vi "Main Responder.vi"(11 "CIFPluginManager in":refnum<class "CIFPluginManager.lvclass">) -> (0 "error out":errorcluster, 3 "Plugin Manager out":refnum<class "CIFPluginManager.lvclass">)   [LabVIEW 2021, in "CIFPluginManager.lvclass"]
uses:
  CIFPluginManager.lvclass
  gRPC/CIF_Manager_client/RPC Messages/cif_common_Empty.ctl
  CIFPluginManager.lvclass/CIFPluginManager.ctl
  <vilib>/Utility/miscctls.llb/LVMapReplaceAction.ctl
  gRPC/CIF_Manager_server/RPC Messages/cif_common_Empty.ctl
  CIFUtilities/CIFLogs/Typedef/Message Type.ctl
  gRPC/CIF_Manager_server/RPC Messages/cif_manager_UnregisterPluginLoaderResponse.ctl
  gRPC/CIF_Manager_server/RPC Messages/cif_manager_PluginTypeReply.ctl
  gRPC/CIF_Manager_server/RPC Messages/cif_manager_PluginType.ctl
  gRPC/CIF_Manager_server/RPC Messages/cif_common_ShortVersion.ctl
  gRPC/CIF_Manager_server/RPC Messages/cif_manager_PluginMetadata.ctl
  gRPC/CIF_Manager_server/RPC Messages/cif_channelcore_Channels.ctl
  gRPC/CIF_Manager_server/RPC Messages/cif_channelcore_Channel.ctl
  gRPC/CIF_Manager_server/RPC Messages/cif_channelcore_ChannelDirection.ctl
  gRPC/CIF_Manager_server/RPC Messages/cif_channelcore_ChannelPattern.ctl
  gRPC/CIF_Manager_server/RPC Messages/cif_manager_ErrorInfoList.ctl
  gRPC/CIF_Manager_server/RPC Messages/cif_manager_ErrorInfo.ctl
  gRPC/CIF_Manager_server/RPC Messages/cif_manager_FileData.ctl
  gRPC/CIF_Manager_server/RPC Messages/cif_manager_PluginInfoArray.ctl
  gRPC/CIF_Manager_server/RPC Messages/cif_manager_PluginInfo.ctl
  gRPC/CIF_Manager_server/RPC Messages/cif_plugincore_StatusData.ctl
  gRPC/CIF_Manager_server/RPC Messages/cif_plugincore_StatusData_PluginState.ctl
  gRPC/CIF_Manager_server/RPC Messages/cif_plugincore_TimingStatistics.ctl
  gRPC/CIF_Manager_server/RPC Messages/cif_common_TimingStats.ctl
  gRPC/CIF_Manager_server/RPC Messages/cif_plugincore_FifoStatistics.ctl
  gRPC/CIF_Manager_server/RPC Messages/cif_plugincore_Error.ctl
  gRPC/CIF_Manager_server/RPC Messages/cif_plugincore_MonitorDoubles.ctl
  gRPC/CIF_Manager_server/RPC Messages/cif_plugincore_MonitorU64.ctl
  gRPC/CIF_Manager_server/RPC Messages/cif_plugincore_MonitorI64.ctl
  gRPC/CIF_Manager_server/RPC Messages/cif_manager_LoaderInfo.ctl
  gRPC/CIF_Manager_server/RPC Messages/cif_manager_LoaderType.ctl
  CIFCore/Common/Typedef/Errors.ctl
  gRPC/CIF_Manager_server/RPC Messages/cif_manager_PluginInfoResponse.ctl
  gRPC/CIF_Manager_server/RPC Messages/cif_common_Status.ctl
  gRPC/CIF_Manager_server/RPC Messages/cif_manager_ClockStatusArray.ctl
  gRPC/CIF_Manager_server/RPC Messages/cif_manager_ClockStatus.ctl
  gRPC/CIF_Manager_server/RPC Messages/cif_manager_ClockConversion.ctl
  gRPC/CIF_Manager_server/RPC Messages/cif_manager_TimePair.ctl
  <vilib>/CIF Foundation/CIF Utilities/Time/Typedef/Timestamp Pair.ctl
  gRPC/CIF_Manager_server/RPC Messages/cif_manager_OrchReturn.ctl
  gRPC/CIF_Manager_server/RPC Messages/cif_manager_DestroyPluginLoaderResponse.ctl
  gRPC/CIF_Manager_server/RPC Messages/Get cif_manager_RegisterData.vi
  gRPC/CIF_Manager_server/RPC Messages/Set cif_common_Empty.vi
  gRPC/CIF_Manager_server/RPC Messages/Get cif_manager_RegisterPluginLoaderRequest.vi
  gRPC/CIF_Manager_server/RPC Messages/Set cif_manager_RegisterPluginLoaderResponse.vi
  gRPC/CIF_Manager_server/RPC Messages/Get cif_manager_UnregisterData.vi
  gRPC/CIF_Manager_server/RPC Messages/Get cif_manager_UnregisterPluginLoaderRequest.vi
  gRPC/CIF_Manager_server/RPC Messages/Set cif_manager_UnregisterPluginLoaderResponse.vi
  gRPC/CIF_Manager_server/RPC Messages/Get cif_manager_QueryTypeSettings.vi
  gRPC/CIF_Manager_server/RPC Messages/Set cif_manager_PluginTypeReply.vi
  gRPC/CIF_Manager_server/RPC Messages/Get cif_channelcore_ChannelFilter.vi
  gRPC/CIF_Manager_server/RPC Messages/Set cif_channelcore_Channels.vi
  gRPC/CIF_Manager_server/RPC Messages/Get cif_common_Empty.vi
  gRPC/CIF_Manager_server/RPC Messages/Set cif_common_Status.vi
  gRPC/CIF_Manager_server/RPC Messages/Get cif_manager_QuerySettings.vi
  gRPC/CIF_Manager_server/RPC Messages/Set cif_manager_ErrorInfoList.vi
  gRPC/CIF_Manager_server/RPC Messages/Set cif_manager_FileData.vi
  gRPC/CIF_Manager_server/RPC Messages/Set cif_manager_PluginInfoArray.vi
  gRPC/CIF_Manager_server/RPC Messages/Get cif_manager_PluginName.vi
  gRPC/CIF_Manager_server/RPC Messages/Set cif_manager_PluginInfoResponse.vi
  <vilib>/CIF Foundation/CIF Utilities/Errors/Append Error Location.vi
  gRPC/CIF_Manager_server/RPC Messages/Set cif_manager_ClockStatusArray.vi
  gRPC/CIF_Manager_server/RPC Messages/Get cif_manager_ClockUpdate.vi
  <vilib>/CIF Foundation/CIF Utilities/Time/SubVIs/Weighted Moving Average for Slope.vi
  <vilib>/CIF Foundation/CIF Utilities/DataTypes/Utilities/Valid Number.vi
  gRPC/CIF_Manager_server/RPC Messages/Get cif_manager_OrchConfig.vi
  gRPC/CIF_Manager_server/RPC Messages/Set cif_manager_OrchReturn.vi
  gRPC/CIF_Manager_server/RPC Messages/Get cif_manager_DestroyPluginLoaderRequest.vi
  gRPC/CIF_Manager_server/RPC Messages/Set cif_manager_DestroyPluginLoaderResponse.vi
  gRPC/CIF_Manager_server/RPC Messages/Get cif_manager_RegisterData.vi/2ed25e12-861d-4677-8ead-ace2906b2041.vi
  gRPC/CIF_Manager_server/RPC Messages/FlatToRichcif_manager_RegisterData.vi
  gRPC/CIF_Manager_server/RPC Messages/Set cif_common_Empty.vi/dcc74a39-081a-4bdd-860b-8ed792803c96.vi
  gRPC/CIF_Manager_server/RPC Messages/RichToFlatcif_common_Empty.vi
  gRPC/CIF_Manager_server/RPC Messages/Get cif_manager_RegisterPluginLoaderRequest.vi/2ed25e12-861d-4677-8ead-ace2906b2041.vi
  gRPC/CIF_Manager_server/RPC Messages/FlatToRichcif_manager_RegisterPluginLoaderRequest.vi
  gRPC/CIF_Manager_server/RPC Messages/Set cif_manager_RegisterPluginLoaderResponse.vi/dcc74a39-081a-4bdd-860b-8ed792803c96.vi
  gRPC/CIF_Manager_server/RPC Messages/RichToFlatcif_manager_RegisterPluginLoaderResponse.vi
  gRPC/CIF_Manager_server/RPC Messages/Get cif_manager_UnregisterData.vi/2ed25e12-861d-4677-8ead-ace2906b2041.vi
  gRPC/CIF_Manager_server/RPC Messages/FlatToRichcif_manager_UnregisterData.vi
  gRPC/CIF_Manager_server/RPC Messages/Get cif_manager_UnregisterPluginLoaderRequest.vi/2ed25e12-861d-4677-8ead-ace2906b2041.vi
  gRPC/CIF_Manager_server/RPC Messages/FlatToRichcif_manager_UnregisterPluginLoaderRequest.vi
  gRPC/CIF_Manager_server/RPC Messages/Set cif_manager_UnregisterPluginLoaderResponse.vi/dcc74a39-081a-4bdd-860b-8ed792803c96.vi
  gRPC/CIF_Manager_server/RPC Messages/RichToFlatcif_manager_UnregisterPluginLoaderResponse.vi
  gRPC/CIF_Manager_server/RPC Messages/Get cif_manager_QueryTypeSettings.vi/2ed25e12-861d-4677-8ead-ace2906b2041.vi
  gRPC/CIF_Manager_server/RPC Messages/FlatToRichcif_manager_QueryTypeSettings.vi
  gRPC/CIF_Manager_server/RPC Messages/Set cif_manager_PluginTypeReply.vi/dcc74a39-081a-4bdd-860b-8ed792803c96.vi
  gRPC/CIF_Manager_server/RPC Messages/RichToFlatcif_manager_PluginTypeReply.vi
  gRPC/CIF_Manager_server/RPC Messages/Get cif_channelcore_ChannelFilter.vi/2ed25e12-861d-4677-8ead-ace2906b2041.vi
  gRPC/CIF_Manager_server/RPC Messages/FlatToRichcif_channelcore_ChannelFilter.vi
  gRPC/CIF_Manager_server/RPC Messages/Set cif_channelcore_Channels.vi/dcc74a39-081a-4bdd-860b-8ed792803c96.vi
  gRPC/CIF_Manager_server/RPC Messages/RichToFlatcif_channelcore_Channels.vi
  gRPC/CIF_Manager_server/RPC Messages/Get cif_common_Empty.vi/2ed25e12-861d-4677-8ead-ace2906b2041.vi
  gRPC/CIF_Manager_server/RPC Messages/FlatToRichcif_common_Empty.vi
  gRPC/CIF_Manager_server/RPC Messages/Set cif_common_Status.vi/dcc74a39-081a-4bdd-860b-8ed792803c96.vi
  gRPC/CIF_Manager_server/RPC Messages/RichToFlatcif_common_Status.vi
  gRPC/CIF_Manager_server/RPC Messages/Get cif_manager_QuerySettings.vi/2ed25e12-861d-4677-8ead-ace2906b2041.vi
  gRPC/CIF_Manager_server/RPC Messages/FlatToRichcif_manager_QuerySettings.vi
  gRPC/CIF_Manager_server/RPC Messages/Set cif_manager_ErrorInfoList.vi/dcc74a39-081a-4bdd-860b-8ed792803c96.vi
  gRPC/CIF_Manager_server/RPC Messages/RichToFlatcif_manager_ErrorInfoList.vi
  gRPC/CIF_Manager_server/RPC Messages/Set cif_manager_FileData.vi/dcc74a39-081a-4bdd-860b-8ed792803c96.vi
  gRPC/CIF_Manager_server/RPC Messages/RichToFlatcif_manager_FileData.vi
  gRPC/CIF_Manager_server/RPC Messages/Set cif_manager_PluginInfoArray.vi/dcc74a39-081a-4bdd-860b-8ed792803c96.vi
  gRPC/CIF_Manager_server/RPC Messages/RichToFlatcif_manager_PluginInfoArray.vi
  gRPC/CIF_Manager_server/RPC Messages/Get cif_manager_PluginName.vi/2ed25e12-861d-4677-8ead-ace2906b2041.vi
  gRPC/CIF_Manager_server/RPC Messages/FlatToRichcif_manager_PluginName.vi
  gRPC/CIF_Manager_server/RPC Messages/Set cif_manager_PluginInfoResponse.vi/dcc74a39-081a-4bdd-860b-8ed792803c96.vi
  gRPC/CIF_Manager_server/RPC Messages/RichToFlatcif_manager_PluginInfoResponse.vi
  gRPC/CIF_Manager_server/RPC Messages/Set cif_manager_ClockStatusArray.vi/dcc74a39-081a-4bdd-860b-8ed792803c96.vi
  gRPC/CIF_Manager_server/RPC Messages/RichToFlatcif_manager_ClockStatusArray.vi
  gRPC/CIF_Manager_server/RPC Messages/Get cif_manager_ClockUpdate.vi/2ed25e12-861d-4677-8ead-ace2906b2041.vi
  gRPC/CIF_Manager_server/RPC Messages/FlatToRichcif_manager_ClockUpdate.vi
  <vilib>/Analysis/3filter.llb/Savitzky-Golay Filter.vi
  <vilib>/Analysis/3filter.llb/Savitzky-Golay Filter (DBL).vi
  gRPC/CIF_Manager_server/RPC Messages/Get cif_manager_OrchConfig.vi/2ed25e12-861d-4677-8ead-ace2906b2041.vi
  gRPC/CIF_Manager_server/RPC Messages/FlatToRichcif_manager_OrchConfig.vi
  gRPC/CIF_Manager_server/RPC Messages/Set cif_manager_OrchReturn.vi/dcc74a39-081a-4bdd-860b-8ed792803c96.vi
  gRPC/CIF_Manager_server/RPC Messages/RichToFlatcif_manager_OrchReturn.vi
  gRPC/CIF_Manager_server/RPC Messages/Get cif_manager_DestroyPluginLoaderRequest.vi/2ed25e12-861d-4677-8ead-ace2906b2041.vi
  gRPC/CIF_Manager_server/RPC Messages/FlatToRichcif_manager_DestroyPluginLoaderRequest.vi
  gRPC/CIF_Manager_server/RPC Messages/Set cif_manager_DestroyPluginLoaderResponse.vi/dcc74a39-081a-4bdd-860b-8ed792803c96.vi
  gRPC/CIF_Manager_server/RPC Messages/RichToFlatcif_manager_DestroyPluginLoaderResponse.vi
  <vilib>/gRPC/LabVIEW gRPC Library/Shared/TranslateGrpcError.vi
  gRPC/CIF_Manager_server/RPC Messages/FlatToRichcif_common_ShortVersion.vi
  gRPC/CIF_Manager_server/RPC Messages/FlatToRichcif_manager_LoaderInfoFull.vi
  gRPC/CIF_Manager_server/RPC Messages/RichToFlatcif_manager_PluginType.vi
  gRPC/CIF_Manager_server/RPC Messages/RichToFlatcif_channelcore_Channel.vi
  gRPC/CIF_Manager_server/RPC Messages/RichToFlatcif_manager_ErrorInfo.vi
  gRPC/CIF_Manager_server/RPC Messages/RichToFlatcif_manager_PluginInfo.vi
  gRPC/CIF_Manager_server/RPC Messages/RichToFlatcif_manager_ClockStatus.vi
  gRPC/CIF_Manager_server/RPC Messages/FlatToRichcif_manager_TimePair.vi
  gRPC/CIF_Manager_server/RPC Messages/RichToFlatcif_common_ShortVersion.vi
  gRPC/CIF_Manager_server/RPC Messages/RichToFlatcif_manager_PluginMetadata.vi
  gRPC/CIF_Manager_server/RPC Messages/RichToFlatcif_plugincore_StatusData.vi
  gRPC/CIF_Manager_server/RPC Messages/RichToFlatcif_manager_LoaderInfo.vi
  gRPC/CIF_Manager_server/RPC Messages/RichToFlatcif_manager_ClockConversion.vi
  gRPC/CIF_Manager_server/RPC Messages/RichToFlatcif_plugincore_TimingStatistics.vi
  gRPC/CIF_Manager_server/RPC Messages/RichToFlatcif_plugincore_FifoStatistics.vi
  gRPC/CIF_Manager_server/RPC Messages/RichToFlatcif_plugincore_Error.vi
  gRPC/CIF_Manager_server/RPC Messages/RichToFlatcif_plugincore_MonitorDoubles.vi
  gRPC/CIF_Manager_server/RPC Messages/RichToFlatcif_plugincore_MonitorU64.vi
  gRPC/CIF_Manager_server/RPC Messages/RichToFlatcif_plugincore_MonitorI64.vi
  gRPC/CIF_Manager_server/RPC Messages/RichToFlatcif_manager_TimePair.vi
  gRPC/CIF_Manager_server/RPC Messages/RichToFlatcif_common_TimingStats.vi
  <vilib>/gRPC/LabVIEW gRPC Library/Server API/Server/Get Server DLL Path.vi
  <vilib>/Utility/error.llb/Error Cluster From Error Code.vi
  <vilib>/gRPC/LabVIEW gRPC Library/Server API/Message Requests/Complete Call.vi
  <vilib>/Analysis/baseanly.llb/Std Deviation and Variance.vi
  <vilib>/Analysis/6fits.llb/Linear Fit.vi
  <vilib>/regexp/Match Regular Expression.xnode
  CIFUtilities/CIFLogs/CIFLogs.lvlib
  gRPC/CIF_Manager_Client_Wrapper/CIFManagerClientWrapper.lvlib
  gRPC/CIF_Manager_client/CIF_Manager_client.lvlib
  gRPC/CIF_Manager_server/RPC Service/Manager/Manager.lvclass
  <vilib>/CIF Foundation/CIF Utilities/Time/Time_CIF_U.lvlib
  CIFCore/Grpc/CIFCoreWrapper/CIFCoreWrapper.lvlib
  CIFUtilities/CIFConfigurationFile/CIF Configuration File.lvlib
  gRPC/CIF_Manager_server/CIF_Manager_server.lvlib
  CIFPluginLoader/gRPC/CIF_Plugin_Loader_Client_Wrapper/CIFPluginLoaderClientWrapper.lvlib
  CIFCore/Common/CIFCoreCommon.lvlib
  CIFUtilities/Scripting/Orchestration/Python/Python Orchestration.lvlib
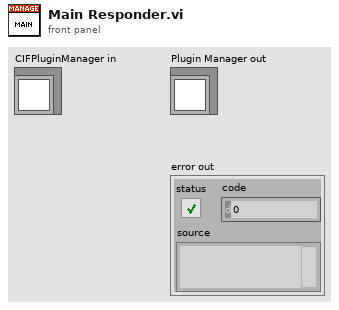
[diagram p1: front panel]
types:
  T1 = typedef "CIF_Manager_client.lvlib/cif_common_Empty.ctl" = cluster{"void":string}
  T2 = typedef "LVMapReplaceAction.ctl" = enum32{"Modify Entry only if found", "Add or Modify Entry", "Delete Entry"}
  T3 = typedef "CIF_Manager_server.lvlib/cif_common_Empty.ctl" = cluster{"void":string}
  T4 = typedef "CIFLogs.lvlib/Message Type.ctl" = enum16{"Error", "Information", "Print Terminal", "Configuration"}
  T5 = typedef "CIF_Manager_server.lvlib/cif_manager_UnregisterPluginLoaderResponse.ctl" = cluster{"void":string}
  T6 = typedef "CIF_Manager_server.lvlib/cif_manager_PluginTypeReply.ctl" = cluster{"plugin_types":T7[]}
  T7 = typedef "CIF_Manager_server.lvlib/cif_manager_PluginType.ctl" = cluster{"plugin_type":string, "plugin_version":T8, "plugin_metadata":T9, "relative_path":string[]}
  T8 = typedef "CIF_Manager_server.lvlib/cif_common_ShortVersion.ctl" = cluster{"major":u32, "minor":u32, "fix":u32}
  T9 = typedef "CIF_Manager_server.lvlib/cif_manager_PluginMetadata.ctl" = cluster{"description":string, "history":string, "author":string}
  T10 = typedef "CIF_Manager_server.lvlib/cif_channelcore_Channels.ctl" = cluster{"channels":T11[]}
  T11 = typedef "CIF_Manager_server.lvlib/cif_channelcore_Channel.ctl" = cluster{"name":string, "direction":T12, "type":string, "custom_config":u8[], "connected":bool, "connected_name":string, "forced":bool, "channel_pattern":T13}
  T12 = typedef "CIF_Manager_server.lvlib/cif_channelcore_ChannelDirection.ctl" = enum32{"CHANNELDIRECTION_UNKNOWN", "CHANNELDIRECTION_PUBLISHER", "CHANNELDIRECTION_SUBSCRIBER"}
  T13 = typedef "CIF_Manager_server.lvlib/cif_channelcore_ChannelPattern.ctl" = enum32{"CHANNELPATTERN_UNKNOWN", "CHANNELPATTERN_TAG", "CHANNELPATTERN_FIFO", "CHANNELPATTERN_MULTIFIFO", "CHANNELPATTERN_BACKPRESSUREFIFO"}
  T14 = typedef "CIF_Manager_server.lvlib/cif_manager_ErrorInfoList.ctl" = cluster{"error_info":T15[]}
  T15 = typedef "CIF_Manager_server.lvlib/cif_manager_ErrorInfo.ctl" = cluster{"error_status":bool, "error_code":i32, "plugin":string, "time":string, "message":string, "location":string}
  T16 = typedef "CIF_Manager_server.lvlib/cif_manager_FileData.ctl" = cluster{"data":string}
  T17 = typedef "CIF_Manager_server.lvlib/cif_manager_PluginInfoArray.ctl" = cluster{"plugin_info":T18[]}
  T18 = typedef "CIF_Manager_server.lvlib/cif_manager_PluginInfo.ctl" = cluster{"plugin_name":string, "plugin_type":string, "grpc_port":i32, "plugin_version":T8, "status":T19, "loader_info":T28}
  T19 = typedef "CIF_Manager_server.lvlib/cif_plugincore_StatusData.ctl" = cluster{"state":T20, "timing_statistics":T21, "fifo_statistics":T23, "error":T24, "monitor_doubles":T25, "monitor_u64s":T26, "monitor_i64s":T27}
  T20 = typedef "CIF_Manager_server.lvlib/cif_plugincore_StatusData_PluginState.ctl" = enum32{"PLUGINSTATE_UNKNOWN", "PLUGINSTATE_CREATING", "PLUGINSTATE_LISTENING", "PLUGINSTATE_RUNNING", "PLUGINSTATE_CLEANINGUP", "PLUGINSTATE_DESTROYING"}
  T21 = typedef "CIF_Manager_server.lvlib/cif_plugincore_TimingStatistics.ctl" = cluster{"period":T22, "wake_error":T22, "execute":T22, "housekeep":T22, "idle":T22, "cleanup":T22, "custom_1":T22, "custom_2":T22}
  T22 = typedef "CIF_Manager_server.lvlib/cif_common_TimingStats.ctl" = cluster{"max":i64, "min":i64, "avg":dbl}
  T23 = typedef "CIF_Manager_server.lvlib/cif_plugincore_FifoStatistics.ctl" = cluster{"from_t0":T22, "from_previous_plugin":T22, "output_error":T22}
  T24 = typedef "CIF_Manager_server.lvlib/cif_plugincore_Error.ctl" = cluster{"status":bool, "code":i32}
  T25 = typedef "CIF_Manager_server.lvlib/cif_plugincore_MonitorDoubles.ctl" = cluster{"double_1":dbl, "double_2":dbl, "double_3":dbl, "double_4":dbl}
  T26 = typedef "CIF_Manager_server.lvlib/cif_plugincore_MonitorU64.ctl" = cluster{"u64_1":u64, "u64_2":u64, "u64_3":u64, "u64_4":u64}
  T27 = typedef "CIF_Manager_server.lvlib/cif_plugincore_MonitorI64.ctl" = cluster{"i64_1":i64, "i64_2":i64, "i64_3":i64, "i64_4":i64}
  T28 = typedef "CIF_Manager_server.lvlib/cif_manager_LoaderInfo.ctl" = cluster{"loader_type":T29, "loader_name":string}
  T29 = typedef "CIF_Manager_server.lvlib/cif_manager_LoaderType.ctl" = enum32{"LOADERTYPE_UNKNOWN", "LOADERTYPE_LABVIEW"}
  T30 = typedef "CIFCoreCommon.lvlib/Errors.ctl" = enum16{"Invalid Clock ID", "Long Sleep", "gRPC Server Not Found", "Config Parse", "Timestamp Wrap", "Delayed Execution", "Duplicate Channel", "Missing Channel", "Incorrect Type", "Flatten Error", "Unflatten Data", "Unique Name", "Plugin Not Found", "Plugin Type Not Found", "Plugin Version Not Found", "Manager Not Found", "Numerical Issue", "Time Jump", "Clock ID Match", "Channel Length", "Plugin Connection", "gRPC Server Connection", "PPL Name Match", "Build", "Config Log Parse", "Plugin Load", "UI Subpanel Load", "Python Name", "Invalid Name", "Unable to Change Ch Buffer", "Failed Kill", "Failed SysExec", "Function Not Implemented", "Load Timeout"}
  T31 = typedef "CIF_Manager_server.lvlib/cif_manager_PluginInfoResponse.ctl" = cluster{"plugin_info":T18, "status":T32}
  T32 = typedef "CIF_Manager_server.lvlib/cif_common_Status.ctl" = cluster{"code":i32, "message":string}
  T33 = typedef "CIF_Manager_server.lvlib/cif_manager_ClockStatusArray.ctl" = cluster{"clocks_status":T34[]}
  T34 = typedef "CIF_Manager_server.lvlib/cif_manager_ClockStatus.ctl" = cluster{"clock_conversion":T35, "error_mean":i64, "error_std_dev":i64}
  T35 = typedef "CIF_Manager_server.lvlib/cif_manager_ClockConversion.ctl" = cluster{"clock_id":u32, "last_reset":i64, "slope":dbl, "offset_pair":T36, "clock_name":string}
  T36 = typedef "CIF_Manager_server.lvlib/cif_manager_TimePair.ctl" = cluster{"system_time":i64, "external_time":i64}
  T37 = typedef "Time_CIF_U.lvlib/Timestamp Pair.ctl" = cluster{"System Time":i64, "External Time":i64}
  T38 = typedef "CIF_Manager_server.lvlib/cif_manager_OrchReturn.ctl" = cluster{"orchestration_script":string, "status":T32}
  T39 = typedef "CIF_Manager_server.lvlib/cif_manager_DestroyPluginLoaderResponse.ctl" = cluster{"status":T32}
  T40 = typedef "grpc-lvsupport-release.lvlib/grpcId.ctl" = u64
  T41 = typedef "CIF_Manager_server.lvlib/cif_manager_RegisterData.ctl" = cluster{"plugin_name":string, "grpc_port":i32, "plugin_version":T8}
  T42 = typedef "CIFPluginManager.lvclass/Plugin Management Data Map.ctl" = map{string, T43}
  T43 = typedef "CIFPluginManager.lvclass/Plugin Management Data.ctl" = cluster{"Unique Name":string, "Plugin Type":string, "gRPC Port":i32, "gRPC ID":T40, "Loader Type":T44, "Loader":string, "Version":T45, "Load Timestamp":i64, "Unload Timestamp":i64, "Unloading":bool, "Ready for removal":bool, "status":T19, "channels":T10}
  T44 = typedef "CIFPluginManager.lvclass/Loader Type.ctl" = enum16{"LabVIEW"}
  T45 = typedef "CIFCoreCommon.lvlib/Version.ctl" = cluster{"Major":i32, "Minor":i32, "Fix":i32, "Build":i32}
  T46 = typedef "CIF_Manager_server.lvlib/cif_manager_RegisterPluginLoaderRequest.ctl" = cluster{"loader_info":T47}
  T47 = typedef "CIF_Manager_server.lvlib/cif_manager_LoaderInfoFull.ctl" = cluster{"loader_type":T29, "loader_name":string, "grpc_port":i32, "pid":u32}
  T48 = typedef "CIFPluginManager.lvclass/Loader Map.ctl" = map{string, T49}
  T49 = typedef "CIFPluginManager.lvclass/Loaders.ctl" = cluster{"Loader Type":T44, "grpc_port":i32, "pid":u32, "gRPC ID":T40, "Load Timestamp":i64, "Unloading":bool, "Ready for removal":bool, "Unload Timestamp":i64}
  T50 = typedef "CIF_Manager_server.lvlib/cif_manager_UnregisterData.ctl" = cluster{"plugin_name":string, "unregister_channels":string[]}
  T51 = typedef "CIF_Manager_server.lvlib/cif_manager_UnregisterPluginLoaderRequest.ctl" = cluster{"loader_name":string}
  T52 = typedef "CIF_Manager_server.lvlib/cif_manager_QueryTypeSettings.ctl" = cluster{"reload":bool}
  T53 = typedef "CIFPluginManager.lvclass/Discovered Plugin Map.ctl" = map{string, T54[]}
  T54 = typedef "CIFPluginManager.lvclass/Discovered Plugin.ctl" = cluster{"Filename":string, "Plugin Type":string, "Qualified name":string, "Version":T45, "Plugin Metadata":T55, "Loader Type":T44, "File Path":string, "Relative Path":string[]}
  T55 = typedef "CIFPluginManager.lvclass/Plugin Metadata.ctl" = cluster{"Description":string, "History":string, "Author":string}
  T56 = typedef "CIF_Manager_server.lvlib/cif_channelcore_ChannelFilter.ctl" = cluster{"name_regex":string, "direction":T12, "direction_filter":bool, "type_regex":string, "forced":bool, "forced_filter":bool}
  T57 = typedef "CIF_Manager_client.lvlib/cif_common_Status.ctl" = cluster{"code":i32, "message":string}
  T58 = typedef "CIF_Manager_server.lvlib/cif_manager_QuerySettings.ctl" = cluster{"query_all":bool}
  T59 = typedef "CIFLogs.lvlib/Error Message.ctl" = cluster{"error":bool, "code":i32, "Message":string, "Location":string, "Plugin":string, "Time":string}
  T60 = typedef "CIFLogs.lvlib/Log Info.ctl" = cluster{"size (bytes)":i64, "Last Timestamp":string}
  T61 = typedef "CIF_Manager_server.lvlib/cif_manager_PluginName.ctl" = cluster{"plugin_name":string}
  T62 = typedef "Time_CIF_U.lvlib/Clock History Map.ctl" = map{u8, T63}
  T63 = typedef "Time_CIF_U.lvlib/Clock History.ctl" = cluster{"System Clock":i64[], "External Clock":i64[], "Last Reset Time":i64, "slope":dbl, "1/slope":dbl, "Offset Pair":T37, "Name":string}
  T64 = typedef "Time_CIF_U.lvlib/Clock Conversion.ctl" = cluster{"ClockID":u8, "Last Reset":i64, "Offset Pair":T37, "Slope":dbl, "1/Slope":dbl, "Name":string}
  T65 = typedef "Time_CIF_U.lvlib/Clock Error Statistics.ctl" = cluster{"mean":i64, "standard deviation":i64}
  T66 = typedef "CIF_Manager_server.lvlib/cif_manager_ClockUpdate.ctl" = cluster{"clock_id":u32, "timestamp_pair":T36, "reinit":bool, "clock_name":string}
  T67 = typedef "CIF_Manager_server.lvlib/cif_manager_OrchConfig.ctl" = cluster{"start_timestamp":u64, "create_file":bool, "orchestration_language":T68, "filename":string, "default_ip":string}
  T68 = typedef "CIF_Manager_server.lvlib/cif_manager_OrchestrationLanguage.ctl" = enum32{"ORCHESTRATIONLANGUAGE_UNKNOWN", "ORCHESTRATIONLANGUAGE_PYTHON"}
  T69 = typedef "CIF_Manager_server.lvlib/cif_manager_DestroyPluginLoaderRequest.ctl" = cluster{"loader_name":string}
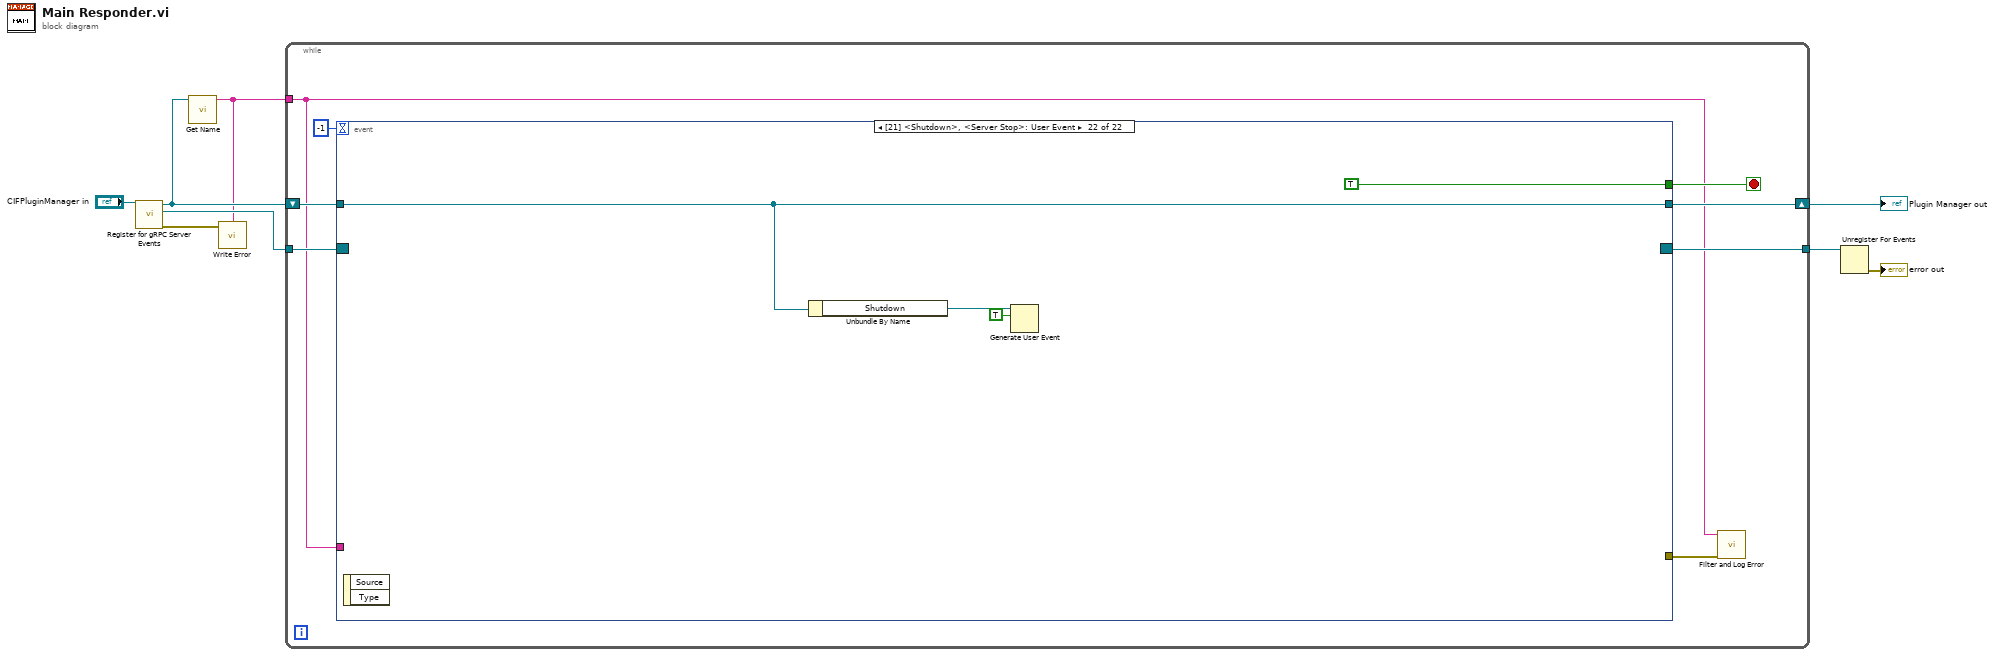
[diagram p0: block diagram]
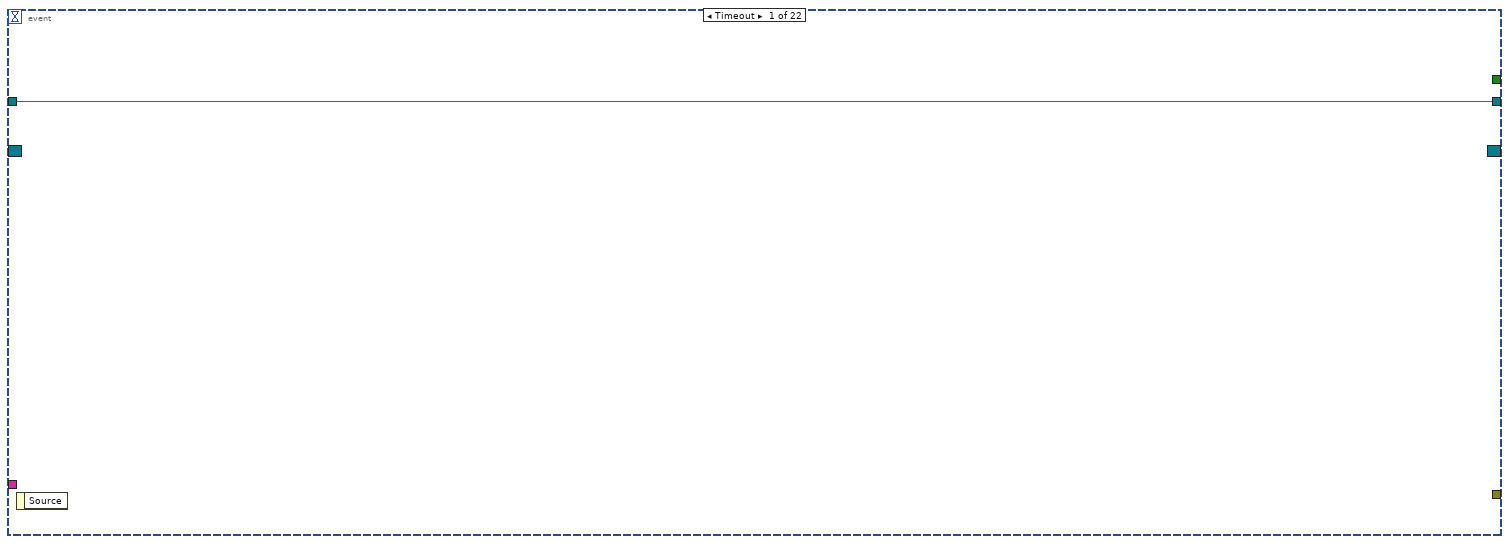
[diagram p2: hidden frame]
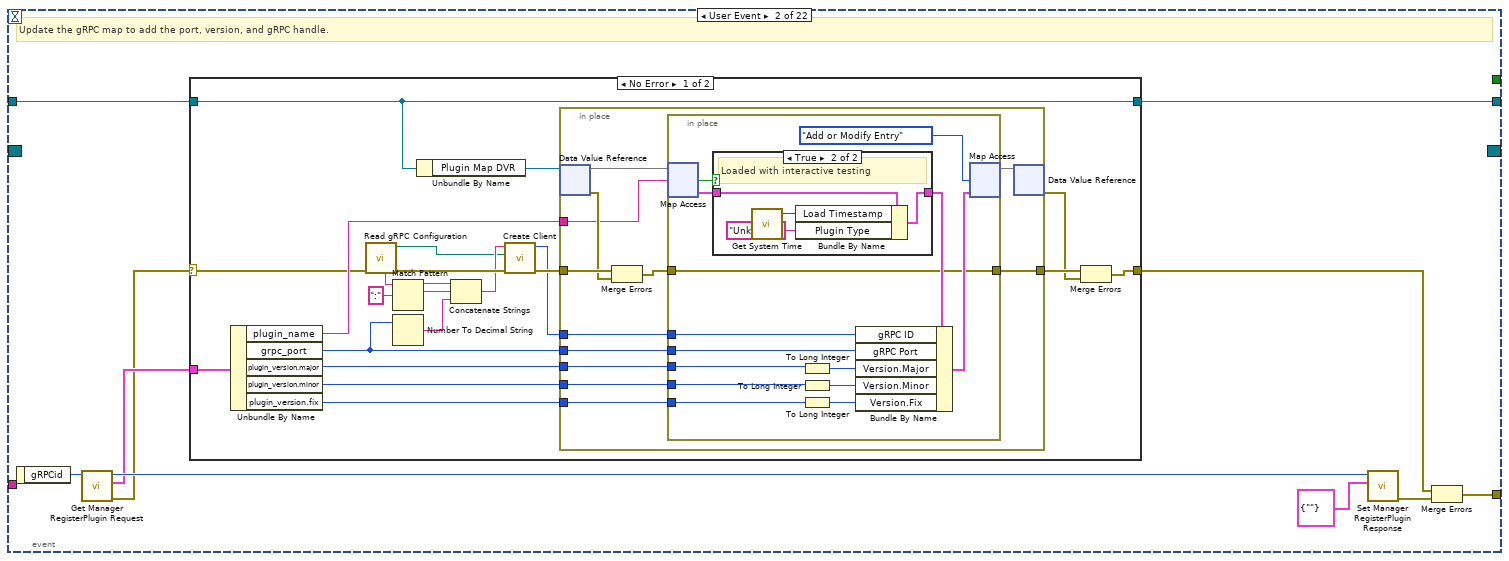
[diagram p3: hidden frame]
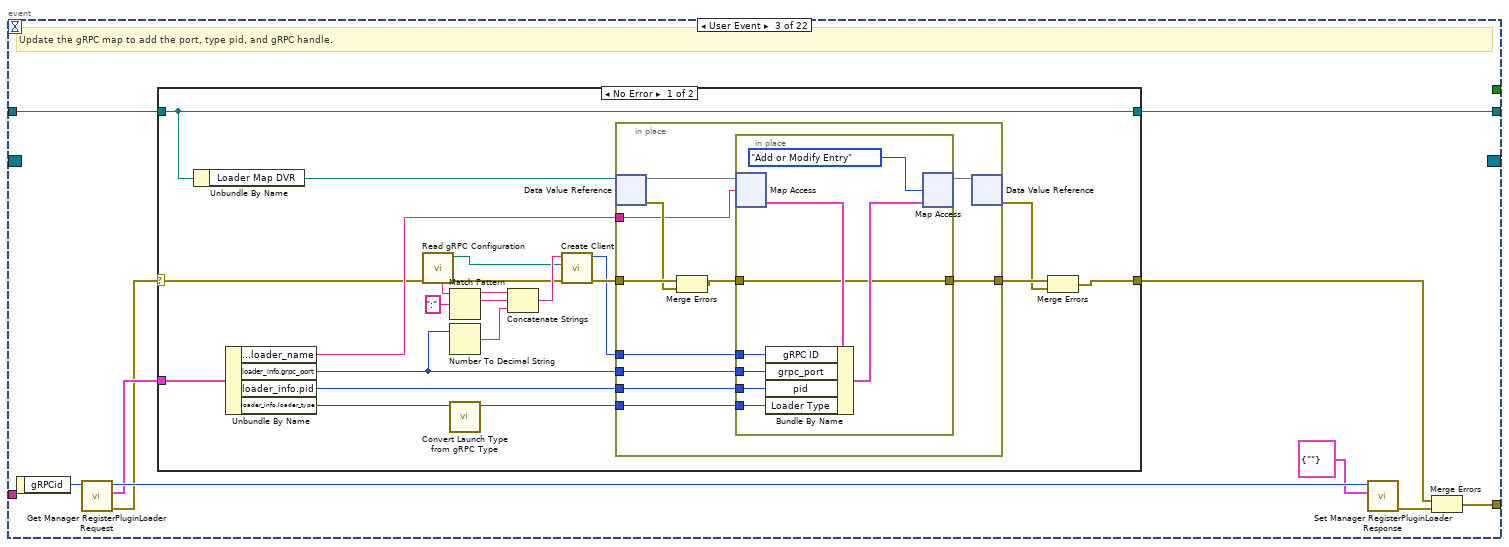
[diagram p6: hidden frame]
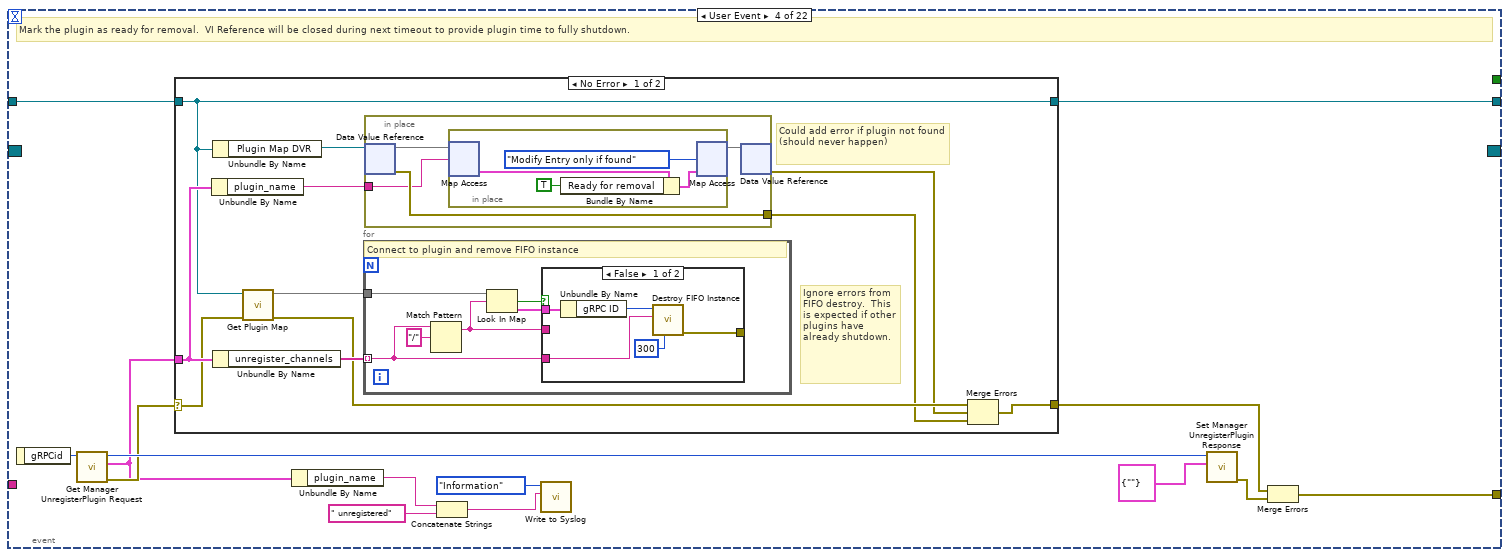
[diagram p8: hidden frame]
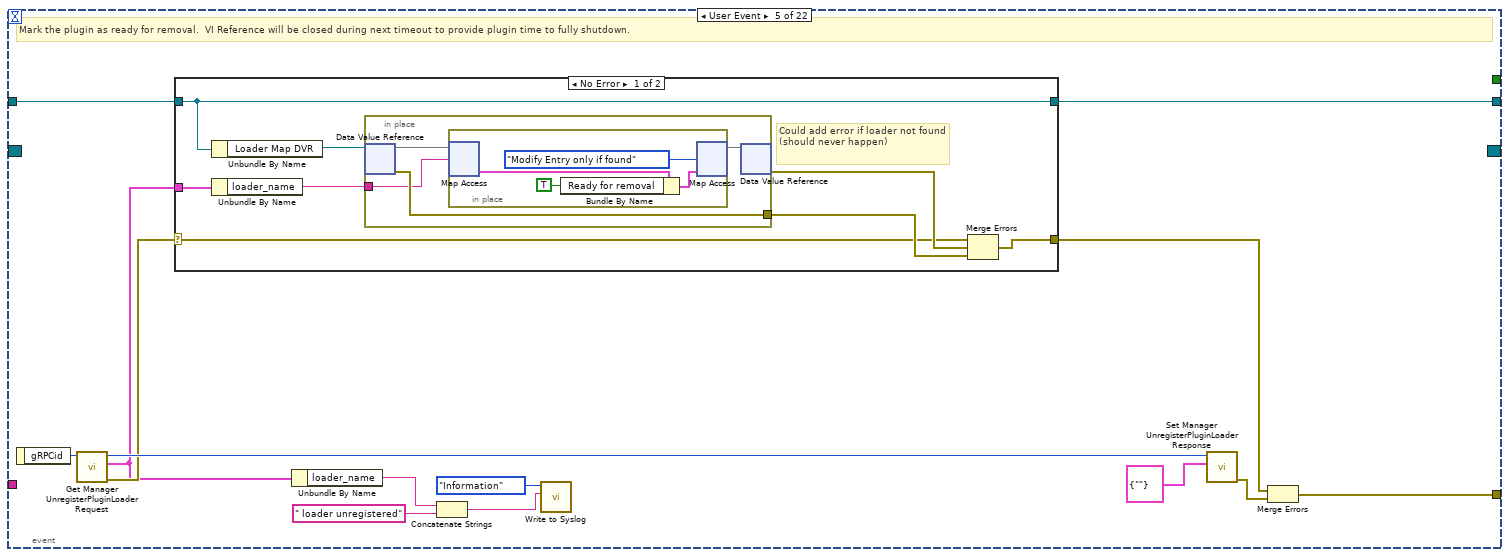
[diagram p11: hidden frame]
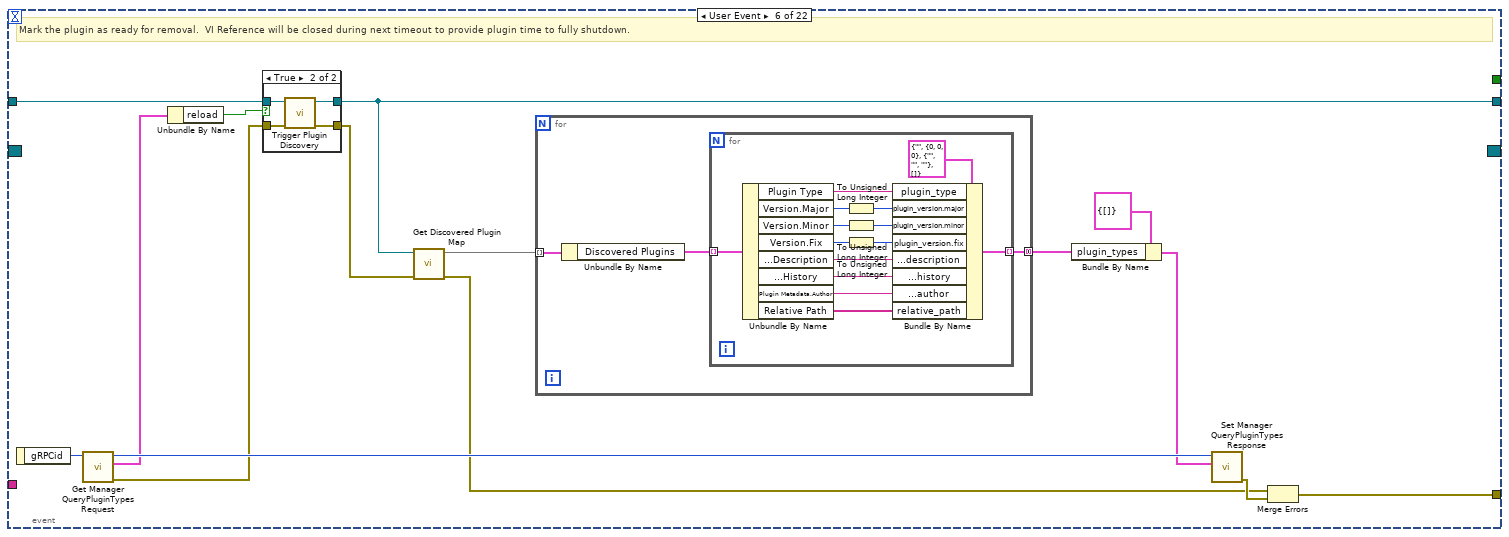
[diagram p13: hidden frame]
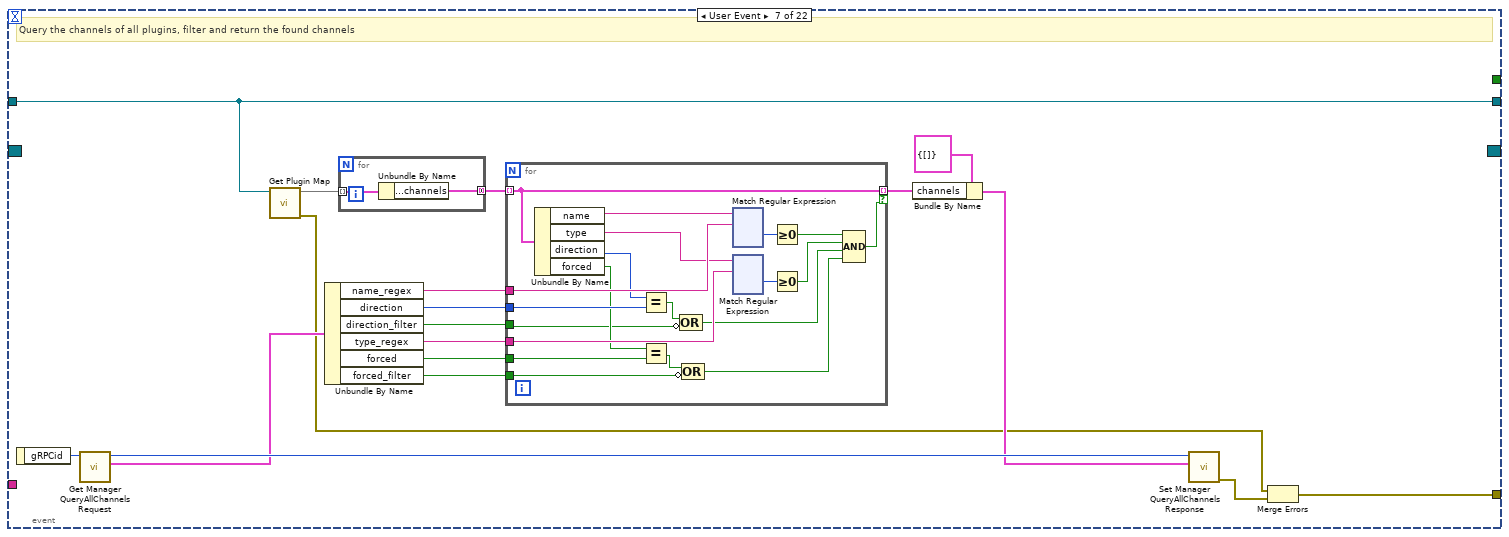
[diagram p15: hidden frame]
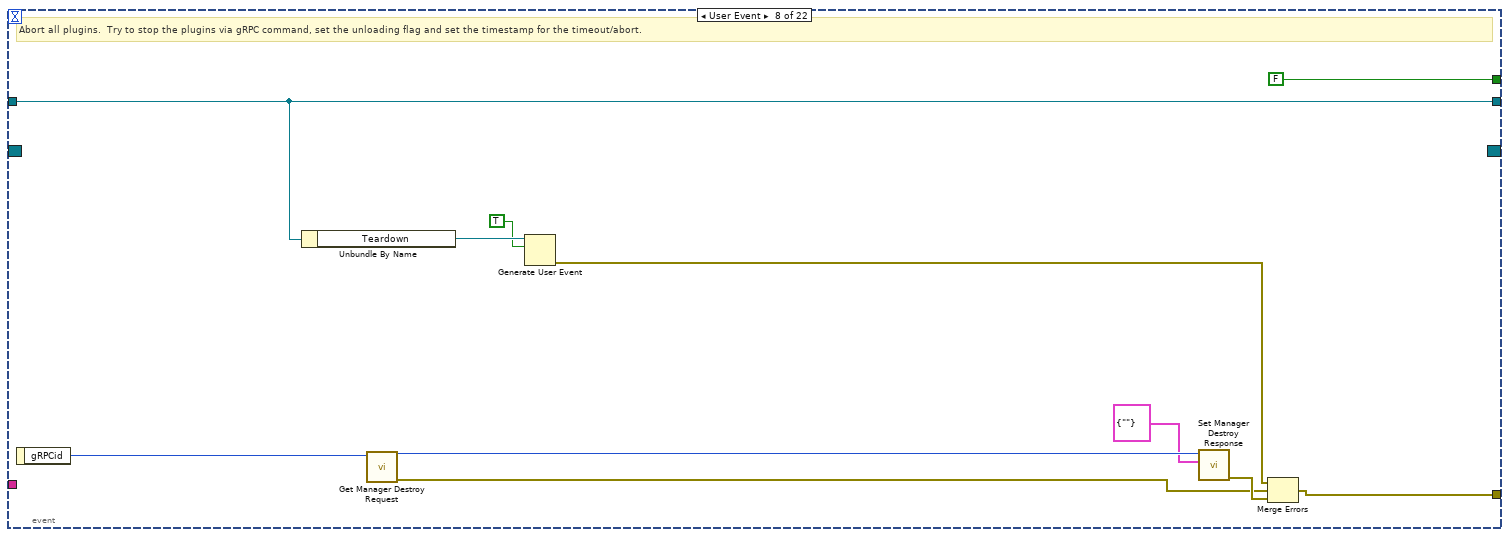
[diagram p16: hidden frame]
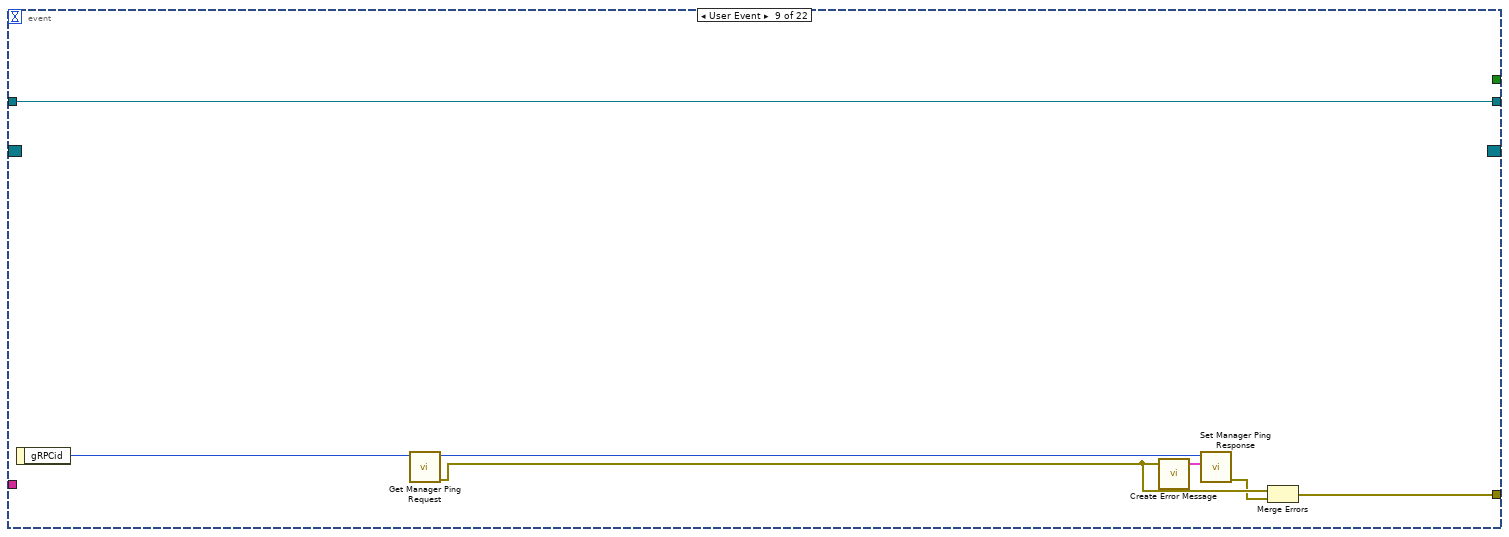
[diagram p17: hidden frame]
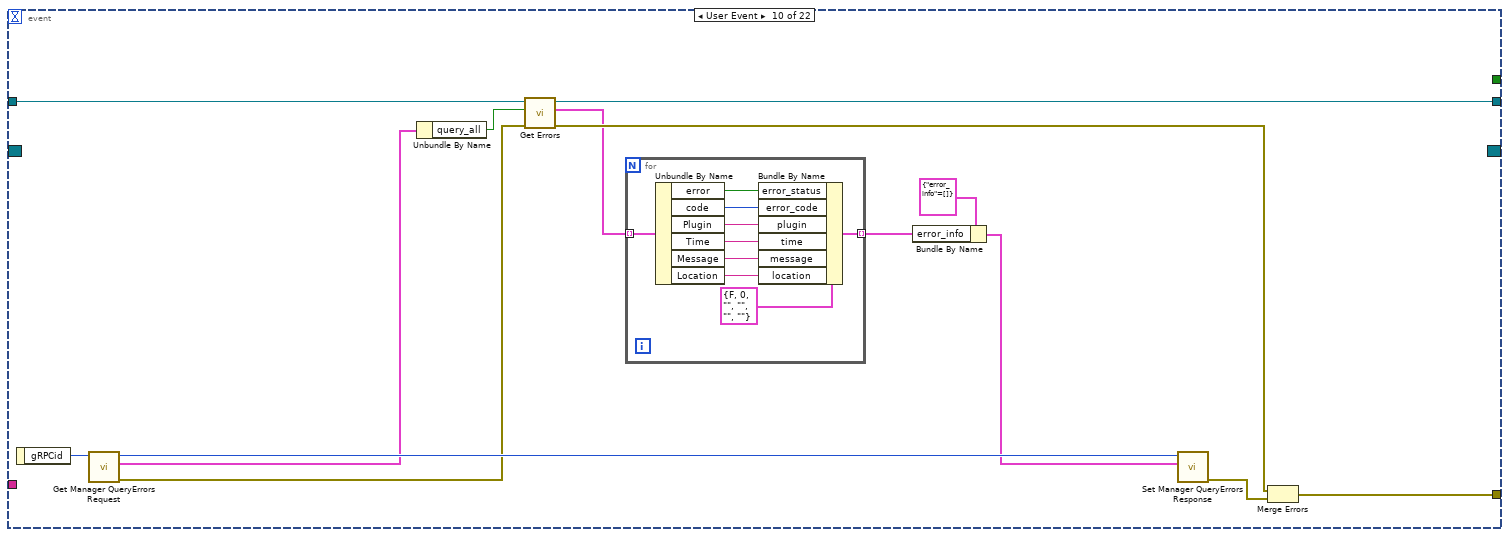
[diagram p18: hidden frame]
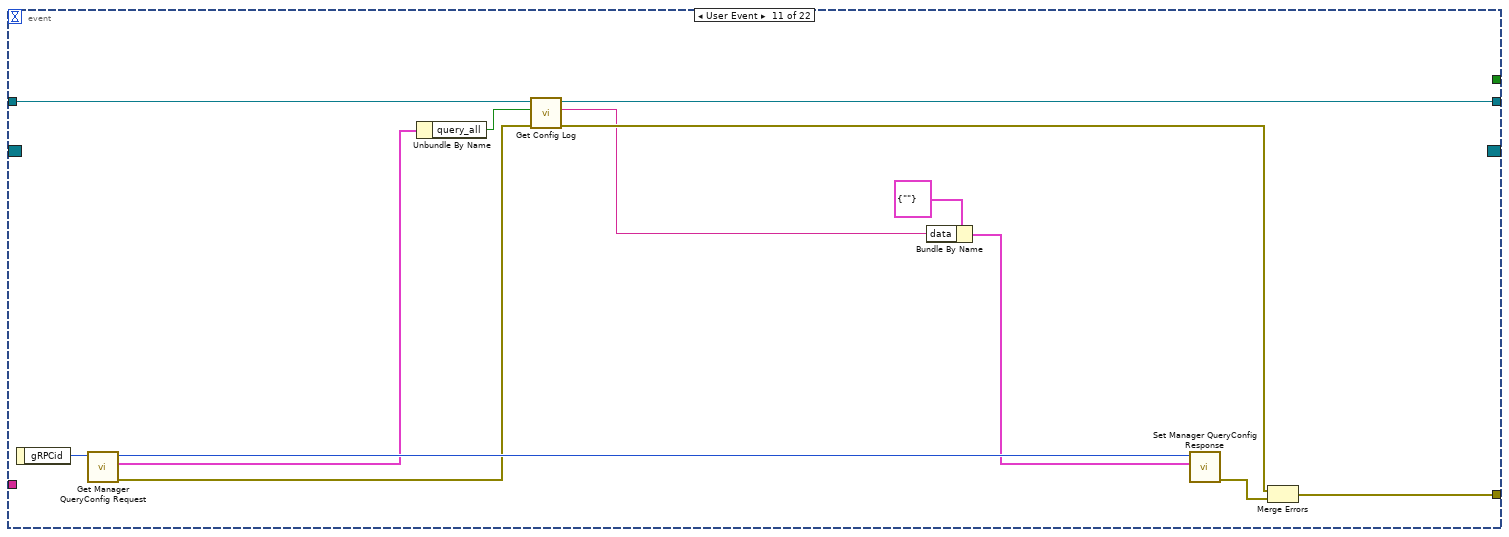
[diagram p19: hidden frame]
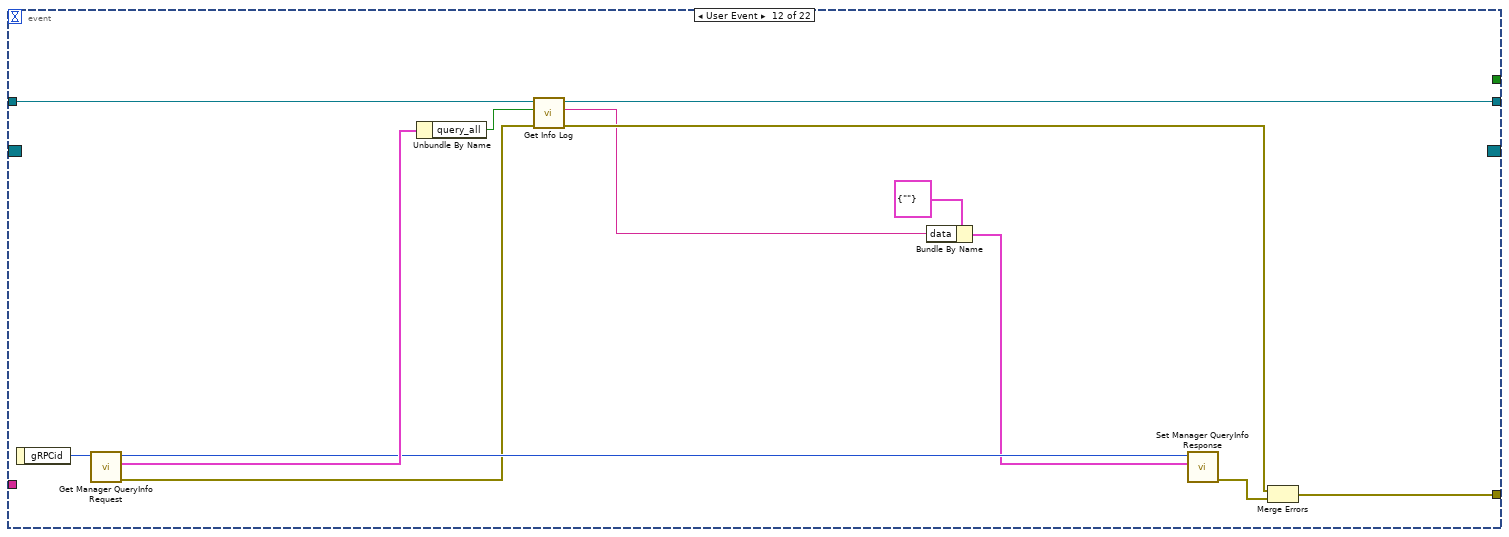
[diagram p20: hidden frame]
diagram:
  n1 = call "Register for gRPC Server Events.vi"("Plugin Manager in"="CIFPluginManager in") -> ("error out"=w8:errorcluster, "Event Registration Refnum"=w3:refnum<event-registration>, "Plugin Manager out"=w2:refnum<class "CIFPluginManager.lvclass">)  [unwired: 8 in]
  n2 = call "Get Name.vi"("CIFPluginManager in"=w2) -> ("Name"=w1:string)  [unwired: 10 in]
  n3 = call "Write Error.vi"("error in (no error)"=w8, "Plugin Name"=w1) -> ()  [unwired: 2 in, 1 out]
  n4 = while {
    tunnel: [w15] -> w6
    shift-right: [w14] -> w5
    shift-left: w2 -> [w16]
    tunnel: w3 -> [w11]
    tunnel: w1 -> [w9]
    stop <- w10 stop-if-true
    n5 = event shown="[21] <Shutdown>, <Server Stop>: User Event" {
      selector: w11 -> [_ _ _ _ _ _ _ _ _ _ _ _ _ _ _ _ _ _ _ _ _ _]
      dyn-events: [_ _ _ _ _ _ _ _ _ _ _ _ _ _ _ _ _ _ _ _ _ _] -> w15
      timeout: -1 -> [_ _ _ _ _ _ _ _ _ _ _ _ _ _ _ _ _ _ _ _ _ _]
      tunnel: w16 -> [w17 w21 w87 w148 w194 w221 w254 w529 w537 w553 w572 w585 w595 w617 w630 w647 w676 w701 w730 w781 w807 w816]
      tunnel: [w17 w19 w85 w147 w193 w217 w254 w529 w537 w549 w569 w581 w594 w616 w628 w647 w676 w701 w730 w780 w807 w816] -> w14
      tunnel: [_ w27 w92 w149 w195 w228 w269 w536 w538 w557 w579 w592 w601 w618 w635 w654 w697 w711 w737 w785 w814 _] -> w13
      tunnel: [_ _ _ _ _ _ _ FALSE _ _ _ _ _ _ _ _ _ _ _ _ _ TRUE] -> w10
      tunnel: w9 -> [_ _ _ _ _ _ _ _ _ _ _ _ _ _ _ _ _ _ _ _ _ _]
      event Timeout {
        n6 = event-data() -> ()  [unwired: 1 in, 1 out]
      }
      event User Event {
        # "Update the gRPC map to add the port, version, and gRPC handle."
        n7 = event-data() -> ("gRPCid"=w25:T40)  [unwired: 1 in]
        n8 = call "Get Manager RegisterPlugin Request.vi"("gRPCid"=w25) -> ("error out"=w20:errorcluster, "Message Data"=w22:T41, "gRPCid out"=w26:T40)  [unwired: 8 in]
        n9 = case shown="No Error" w20 {
          selector: w20 -> [w33 w81]
          tunnel: w22 -> [w44 _]
          tunnel: w21 -> [w49 w82]
          tunnel: [w49 w82] -> w19
          tunnel: [w45 w81] -> w18
          frame No Error {
            n10 = Unbundle By Name(w44) -> ("plugin_name"=w43:string, "grpc_port"=w31:i32, "plugin_version.major"=w42:u32, "plugin_version.minor"=w41:u32, "plugin_version.fix"=w40:u32)
            n11 = call "Read gRPC Configuration.vi"("error in"=w33) -> ("error out"=w35:errorcluster, "Server Certificate File (.crt)"=w28:path, "Local Manager Address"=w36:string)  [unwired: 5 in, 3 out]
            n12 = Match Pattern(string=w36, regular expression=":") -> (before substring=w37:string, match substring=w38:string)  [unwired: 1 in, 2 out]
            n13 = Number To Decimal String(number=w31) -> (decimal integer string=w39:string)  [unwired: 1 in]
            n14 = Unbundle By Name(w49) -> ("Plugin Map DVR"=w48:refnum<data-value>)
            n15 = Concatenate Strings(w37, w38, w39) -> (w30:string)
            n16 = call "Create Client.vi"("error in"=w35, "Server Certificate File (.crt)"=w28, "address"=w30) -> ("error out"=w32:errorcluster, "gRPC ID Out"=w29:T40)  [unwired: 7 in]
            n17 = in-place {
              in-place-border: w32 -> [w59]
              in-place-border: [w61] -> w47
              in-place-border: w43 -> [w55]
              in-place-border: w31 -> [w54]
              in-place-border: w42 -> [w53]
              in-place-border: w41 -> [w52]
              in-place-border: w40 -> [w51]
              in-place-border: w29 -> [w50]
              n18 = in-place-dvr #1(w48) -> (w60:T42, w58:errorcluster)
              n19 = Merge Errors(w59, w58) -> (w57:errorcluster)
              n20 = in-place {
                in-place-border: w57 -> [w63]
                in-place-border: [w63] -> w61
                in-place-border: w54 -> [w67]
                in-place-border: w53 -> [w66]
                in-place-border: w52 -> [w65]
                in-place-border: w51 -> [w64]
                in-place-border: w50 -> [w62]
                n21 = in-place-map #2(w60, w55) -> (w69:T43, w70:bool)  [unwired: 1 in]
                n22 = case shown="True" w70 {
                  tunnel: w69 -> [w76 w80]
                  tunnel: [w76 w79] -> w68
                  frame False {
                  }
                  frame True {
                    # "Loaded with interactive testing"
                    n23 = call <vilib>:"Get System Time.vi"() -> ("Time (ns)"=w77:i64)  [unwired: 5 in]
                    n24 = Bundle By Name(cluster=w80, "Load Timestamp"=w77, "Plugin Type"="Unknown") -> (w79:T43)
                  }
                }
                n25 = To Long Integer(number=w66) -> (32bit integer=w73:i32)
                n26 = To Long Integer(number=w65) -> (32bit integer=w72:i32)
                n27 = To Long Integer(number=w64) -> (32bit integer=w71:i32)
                n28 = Bundle By Name(cluster=w68, "gRPC ID"=w62, "gRPC Port"=w67, "Version.Major"=w73, "Version.Minor"=w72, "Version.Fix"=w71) -> (w75:T43)
                n29 = in-place-map #2(w75, LVMapReplaceAction."Add or Modify Entry" ("action")) -> (w56:T42)  [unwired: 2 out]
              }
              n30 = in-place-dvr #1(w56) -> (w46:errorcluster)  [unwired: 1 out]
            }
            n31 = Merge Errors(w47, w46) -> (w45:errorcluster)
          }
          frame Error {
          }
        }
        n32 = call "Set Manager RegisterPlugin Response.vi"("Message Data"=T1 {"void"=""}, "gRPCid in"=w26) -> ("error out"=w24:errorcluster)  [unwired: 9 in]
        n33 = Merge Errors(w18, w24) -> (w27:errorcluster)
      }
      event User Event {
        # "Update the gRPC map to add the port, type pid, and gRPC handle."
        n34 = event-data() -> ("gRPCid"=w90:T40)  [unwired: 1 in]
        n35 = call "Get Manager RegisterPluginLoader Request.vi"("gRPCid"=w90) -> ("error out"=w86:errorcluster, "Message Data"=w88:T46, "gRPCid out"=w91:T40)  [unwired: 8 in]
        n36 = case shown="No Error" w86 {
          selector: w86 -> [w98 w134]
          tunnel: w88 -> [w109 _]
          tunnel: w87 -> [w114 w135]
          tunnel: [w114 w135] -> w85
          tunnel: [w110 w134] -> w84
          frame No Error {
            n37 = Unbundle By Name(w114) -> ("Loader Map DVR"=w113:refnum<data-value>)
            n38 = Unbundle By Name(w109) -> ("loader_info.loader_name"=w108:string, "loader_info.grpc_port"=w96:i32, "loader_info.pid"=w107:u32, "loader_info.loader_type"=w94:T29)
            n39 = call "Read gRPC Configuration.vi"("error in"=w98) -> ("error out"=w100:errorcluster, "Server Certificate File (.crt)"=w105:path, "Local Manager Address"=w101:string)  [unwired: 5 in, 3 out]
            n40 = Match Pattern(string=w101, regular expression=":") -> (before substring=w102:string, match substring=w103:string)  [unwired: 1 in, 2 out]
            n41 = Number To Decimal String(number=w96) -> (decimal integer string=w104:string)  [unwired: 1 in]
            n42 = call "Convert Launch Type from gRPC Type.vi"("Loader Type"=w94) -> ("Loader Type"=w93:T44)  [unwired: 9 in, 1 out]
            n43 = Concatenate Strings(w102, w103, w104) -> (w106:string)
            n44 = call "Create Client.vi"("error in"=w100, "Server Certificate File (.crt)"=w105, "address"=w106) -> ("error out"=w97:errorcluster, "gRPC ID Out"=w95:T40)  [unwired: 7 in]
            n45 = in-place {
              in-place-border: w97 -> [w123]
              in-place-border: [w125] -> w112
              in-place-border: w108 -> [w119]
              in-place-border: w96 -> [w118]
              in-place-border: w107 -> [w117]
              in-place-border: w93 -> [w116]
              in-place-border: w95 -> [w115]
              n46 = in-place-dvr #3(w113) -> (w124:T48, w122:errorcluster)
              n47 = Merge Errors(w123, w122) -> (w121:errorcluster)
              n48 = in-place {
                in-place-border: w121 -> [w130]
                in-place-border: [w130] -> w125
                in-place-border: w118 -> [w129]
                in-place-border: w117 -> [w128]
                in-place-border: w116 -> [w127]
                in-place-border: w115 -> [w126]
                n49 = in-place-map #4(w124, w119) -> (w131:T49)  [unwired: 1 in, 1 out]
                n50 = Bundle By Name(cluster=w131, "gRPC ID"=w126, "grpc_port"=w129, "pid"=w128, "Loader Type"=w127) -> (w133:T49)
                n51 = in-place-map #4(w133, LVMapReplaceAction."Add or Modify Entry" ("action")) -> (w120:T48)  [unwired: 2 out]
              }
              n52 = in-place-dvr #3(w120) -> (w111:errorcluster)  [unwired: 1 out]
            }
            n53 = Merge Errors(w112, w111) -> (w110:errorcluster)
          }
          frame Error {
          }
        }
        n54 = call "Set Manager RegisterPluginLoader Response.vi"("Message Data"=T3 {"void"=""}, "gRPCid in"=w91) -> ("error out"=w89:errorcluster)  [unwired: 9 in]
        n55 = Merge Errors(w84, w89) -> (w92:errorcluster)
      }
      event User Event {
        # "Mark the plugin as ready for removal.  VI Reference will be closed during next timeout to provide plugin time to fully shutdown."
        n56 = event-data() -> ("gRPCid"=w146:T40)  [unwired: 1 in]
        n57 = call "Get Manager UnregisterPlugin Request.vi"("gRPCid"=w146) -> ("error out"=w142:errorcluster, "Message Data"=w139:T50, "gRPCid out"=w145:T40)  [unwired: 8 in]
        n58 = case shown="No Error" w142 {
          selector: w142 -> [w158 w180]
          tunnel: w139 -> [w160 _]
          tunnel: w148 -> [w156 w181]
          tunnel: [w156 w181] -> w147
          tunnel: [w151 w180] -> w141
          frame No Error {
            # "Could add error if plugin not found (should never happen)"
            # "Ignore errors from FIFO destroy.  This is expected if other plugins have already shutdown."
            n59 = Unbundle By Name(w160) -> ("plugin_name"=w150:string)
            n60 = Unbundle By Name(w156) -> ("Plugin Map DVR"=w155:refnum<data-value>)
            n61 = Unbundle By Name(w160) -> ("unregister_channels"=w159:string[])
            n62 = call "Get Plugin Map.vi"("error in (no error)"=w158, "CIFPluginManager in"=w156) -> ("error out"=w154:errorcluster, "Plugin Map"=w157:T42)  [unwired: 8 in]
            n63 = for {
              tunnel: w159 -> [w174] mode=indexing
              tunnel: w157 -> [w169]
              # "Connect to plugin and remove FIFO instance"
              n64 = Match Pattern(string=w174, regular expression="/") -> (before substring=w170:string)  [unwired: 1 in, 3 out]
              n65 = Look In Map(map=w169, key=w170) -> (key not found?=w172:bool, value=w171:T43)  [unwired: 1 in]
              n66 = case shown="False" w172 {
                tunnel: w171 -> [w179 _]
                tunnel: w174 -> [w177 _]
                tunnel: w170 -> [_ _]
                tunnel: [w176 _] -> _
                frame False {
                  n67 = Unbundle By Name(w179) -> ("gRPC ID"=w178:T40)
                  n68 = call "Destroy FIFO Instance.vi"("timeout (ms)"=300, "publisher_instance_name"=w177, "gRPC ID"=w178) -> ("error out"=w176:errorcluster)  [unwired: 7 in, 1 out]
                }
                frame True {
                }
              }
            }
            n69 = in-place {
              in-place-border: [w164] -> w153
              in-place-border: w150 -> [w161]
              n70 = in-place-dvr #5(w155) -> (w163:T42, w164:errorcluster)
              n71 = in-place {
                n72 = in-place-map #6(w163, w161) -> (w167:T43)  [unwired: 1 in, 1 out]
                n73 = Bundle By Name(cluster=w167, "Ready for removal"=TRUE) -> (w166:T43)
                n74 = in-place-map #6(w166, LVMapReplaceAction."Modify Entry only if found" ("action")) -> (w162:T42)  [unwired: 2 out]
              }
              n75 = in-place-dvr #5(w162) -> (w152:errorcluster)  [unwired: 1 out]
            }
            n76 = Merge Errors(w154, w152, w153) -> (w151:errorcluster)
          }
          frame Error {
          }
        }
        n77 = Unbundle By Name(w139) -> ("plugin_name"=w137:string)
        n78 = Concatenate Strings(w137, " unregistered" ("message")) -> (w138:string)
        n79 = call "Write to Syslog.vi"("message"=w138, "CIF Message Type"=Message_Type."Information") -> ()  [unwired: 9 in, 1 out]
        n80 = call "Set Manager UnregisterPlugin Response.vi"("Message Data"=T1 {"void"=""}, "gRPCid in"=w145) -> ("error out"=w144:errorcluster)  [unwired: 9 in]
        n81 = Merge Errors(w141, w144) -> (w149:errorcluster)
      }
      event User Event {
        # "Mark the plugin as ready for removal.  VI Reference will be closed during next timeout to provide plugin time to fully shutdown."
        n82 = event-data() -> ("gRPCid"=w192:T40)  [unwired: 1 in]
        n83 = call "Get Manager UnregisterPluginLoader Request.vi"("gRPCid"=w192) -> ("error out"=w189:errorcluster, "Message Data"=w186:T51, "gRPCid out"=w191:T40)  [unwired: 8 in]
        n84 = case shown="No Error" w189 {
          selector: w189 -> [w196 w212]
          tunnel: w186 -> [w203 _]
          tunnel: w194 -> [w202 w213]
          tunnel: [w202 w213] -> w193
          tunnel: [w198 w212] -> w188
          frame No Error {
            # "Could add error if loader not found (should never happen)"
            n85 = Unbundle By Name(w202) -> ("Loader Map DVR"=w201:refnum<data-value>)
            n86 = Unbundle By Name(w203) -> ("loader_name"=w197:string)
            n87 = in-place {
              in-place-border: [w207] -> w200
              in-place-border: w197 -> [w204]
              n88 = in-place-dvr #7(w201) -> (w206:T48, w207:errorcluster)
              n89 = in-place {
                n90 = in-place-map #8(w206, w204) -> (w210:T49)  [unwired: 1 in, 1 out]
                n91 = Bundle By Name(cluster=w210, "Ready for removal"=TRUE) -> (w209:T49)
                n92 = in-place-map #8(w209, LVMapReplaceAction."Modify Entry only if found" ("action")) -> (w205:T48)  [unwired: 2 out]
              }
              n93 = in-place-dvr #7(w205) -> (w199:errorcluster)  [unwired: 1 out]
            }
            n94 = Merge Errors(w196, w199, w200) -> (w198:errorcluster)
          }
          frame Error {
          }
        }
        n95 = Unbundle By Name(w186) -> ("loader_name"=w184:string)
        n96 = Concatenate Strings(w184, " loader unregistered" ("message")) -> (w185:string)
        n97 = call "Write to Syslog.vi"("message"=w185, "CIF Message Type"=Message_Type."Information") -> ()  [unwired: 9 in, 1 out]
        n98 = call "Set Manager UnregisterPluginLoader Response.vi"("Message Data"=T5 {"void"=""}, "gRPCid in"=w191) -> ("error out"=w190:errorcluster)  [unwired: 9 in]
        n99 = Merge Errors(w188, w190) -> (w195:errorcluster)
      }
      event User Event {
        # "Mark the plugin as ready for removal.  VI Reference will be closed during next timeout to provide plugin time to fully shutdown."
        n100 = event-data() -> ("gRPCid"=w227:T40)  [unwired: 1 in]
        n101 = call "Get Manager QueryPluginTypes Request.vi"("gRPCid"=w227) -> ("error out"=w220:errorcluster, "Message Data"=w219:T52, "gRPCid out"=w226:T40)  [unwired: 8 in]
        n102 = Unbundle By Name(w219) -> ("reload"=w218:bool)
        n103 = case shown="True" w218 {
          tunnel: w221 -> [w230 w234]
          tunnel: [w230 w233] -> w217
          tunnel: [w229 w232] -> w216
          tunnel: w220 -> [w229 w231]
          frame False {
          }
          frame True {
            n104 = call "Trigger Plugin Discovery.vi"("error in (no error)"=w231, "CIFPluginManager in"=w234) -> ("error out"=w232:errorcluster, "CIFPluginManager out"=w233:refnum<class "CIFPluginManager.lvclass">)  [unwired: 8 in]
          }
        }
        n105 = call "Get Discovered Plugin Map.vi"("error in (no error)"=w216, "CIFPluginManager in"=w217) -> ("error out"=w214:errorcluster, "Discovered Plugins"=w215:T53)  [unwired: 8 in]
        n106 = for {
          tunnel: w215 -> [w237] mode=indexing
          tunnel: [w235] -> w223 mode=concatenating
          n107 = Unbundle By Name(w237) -> ("Discovered Plugins"=w236:T54[])
          n108 = for {
            tunnel: w236 -> [w251] mode=indexing
            tunnel: [w245] -> w235 mode=indexing
            n109 = Unbundle By Name(w251) -> ("Plugin Type"=w246:string, "Version.Major"=w247:i32, "Version.Minor"=w248:i32, "Version.Fix"=w249:i32, "Plugin Metadata.Description"=w244:string, "Plugin Metadata.History"=w243:string, "Plugin Metadata.Author"=w242:string, "Relative Path"=w238:string[])
            n110 = To Unsigned Long Integer(number=w247) -> (unsigned 32bit integer=w239:u32)
            n111 = To Unsigned Long Integer(number=w248) -> (unsigned 32bit integer=w240:u32)
            n112 = To Unsigned Long Integer(number=w249) -> (unsigned 32bit integer=w241:u32)
            n113 = Bundle By Name(cluster=T7 {"plugin_type"="", "plugin_version"={"major"=0, "minor"=0, "fix"=0}, "plugin_metadata"={"description"="", "history"="", "author"=""}, "relative_path"=[]} ("cif_manager_PluginType"), "plugin_type"=w246, "plugin_version.major"=w239, "plugin_version.minor"=w240, "plugin_version.fix"=w241, "plugin_metadata.description"=w244, "plugin_metadata.history"=w243, "plugin_metadata.author"=w242, "relative_path"=w238) -> (w245:T7)
          }
        }
        n114 = Bundle By Name(cluster=T6 {"plugin_types"=[]} ("Message Data"), "plugin_types"=w223) -> (w222:T6)
        n115 = call "Set Manager QueryPluginTypes Response.vi"("Message Data"=w222, "gRPCid in"=w226) -> ("error out"=w225:errorcluster)  [unwired: 9 in]
        n116 = Merge Errors(w214, w225) -> (w228:errorcluster)
      }
      event User Event {
        # "Query the channels of all plugins, filter and return the found channels"
        n117 = event-data() -> ("gRPCid"=w267:T40)  [unwired: 1 in]
        n118 = call "Get Manager QueryAllChannels Request.vi"("gRPCid"=w267) -> ("Message Data"=w264:T56, "gRPCid out"=w268:T40)  [unwired: 8 in, 1 out]
        n119 = call "Get Plugin Map.vi"("CIFPluginManager in"=w254) -> ("error out"=w252:errorcluster, "Plugin Map"=w253:T42)  [unwired: 9 in]
        n120 = Unbundle By Name(w264) -> ("name_regex"=w263:string, "direction"=w262:T12, "direction_filter"=w261:bool, "type_regex"=w260:string, "forced"=w259:bool, "forced_filter"=w258:bool)
        n121 = for {
          tunnel: w253 -> [w525] mode=indexing
          tunnel: [w524] -> w265 mode=concatenating
          n122 = Unbundle By Name(w525) -> ("Plugin Management Data.channels.channels"=w524:T11[])
        }
        n123 = for {
          tunnel: w265 -> [w289] mode=indexing
          tunnel: [w289] -> w256 mode=indexing if=w270
          tunnel: w263 -> [w287]
          tunnel: w262 -> [w281]
          tunnel: w261 -> [w277]
          tunnel: w260 -> [w285]
          tunnel: w259 -> [w279]
          tunnel: w258 -> [w276]
          n124 = Unbundle By Name(w289) -> ("name"=w288:string, "type"=w286:string, "direction"=w282:T12, "forced"=w280:bool)
          n125 = Equal?(x=w282, y=w281) -> (x = y?=w278:bool)
          n126 = Equal?(x=w280, y=w279) -> (x = y?=w275:bool)
          n127 = Compound Arithmetic op=OR(w278, invert w277) -> (w272:bool)
          n128 = Compound Arithmetic op=OR(w275, invert w276) -> (w271:bool)
          n129 = xnode "Match Regular Expression"("input string"=w288, "regular expression"=w287) -> ("offset past match"=w284:i32)  [unwired: 4 in, 4 out]
          n130 = xnode "Match Regular Expression"("input string"=w286, "regular expression"=w285) -> ("offset past match"=w283:i32)  [unwired: 4 in, 4 out]
          n131 = Greater Or Equal To 0?(x=w284) -> (x >= 0?=w274:bool)
          n132 = Greater Or Equal To 0?(x=w283) -> (x >= 0?=w273:bool)
          n133 = Compound Arithmetic op=AND(w274, w273, w272, w271) -> (w270:bool)
        }
        n134 = Bundle By Name(cluster=T10 {"channels"=[]} ("Message Data"), "channels"=w256) -> (w255:T10)
        n135 = call "Set Manager QueryAllChannels Response.vi"("Message Data"=w255, "gRPCid in"=w268) -> ("error out"=w266:errorcluster)  [unwired: 9 in]
        n136 = Merge Errors(w252, w266) -> (w269:errorcluster)
      }
      event User Event {
        # "Abort all plugins.  Try to stop the plugins via gRPC command, set the unloading flag and set the timestamp for the timeout/abort."
        n137 = event-data() -> ("gRPCid"=w535:T40)  [unwired: 1 in]
        n138 = Unbundle By Name(w529) -> ("Teardown"=w528:refnum<user-event>)
        n139 = call "Get Manager Destroy Request.vi"("gRPCid"=w535) -> ("error out"=w530:errorcluster, "gRPCid out"=w534:T40)  [unwired: 8 in, 1 out]
        n140 = Generate User Event(user event=w528, event data cluster=TRUE ("event data")) -> (error out=w526:errorcluster)  [unwired: 2 in, 1 out]
        n141 = call "Set Manager Destroy Response.vi"("Message Data"=T1 {"void"=""}, "gRPCid in"=w534) -> ("error out"=w533:errorcluster)  [unwired: 9 in]
        n142 = Merge Errors(w526, w530, w533) -> (w536:errorcluster)
      }
      event User Event {
        n143 = event-data() -> ("gRPCid"=w543:T40)  [unwired: 1 in]
        n144 = call "Get Manager Ping Request.vi"("gRPCid"=w543) -> ("error out"=w540:errorcluster, "gRPCid out"=w542:T40)  [unwired: 8 in, 1 out]
        n145 = call "Create Error Message.vi"("error in (no error)"=w540) -> ("Error Message"=w541:T57)  [unwired: 3 in]
        n146 = call "Set Manager Ping Response.vi"("Message Data"=w541, "gRPCid in"=w542) -> ("error out"=w539:errorcluster)  [unwired: 9 in]
        n147 = Merge Errors(w540, w539) -> (w538:errorcluster)
      }
      event User Event {
        n148 = event-data() -> ("gRPCid"=w556:T40)  [unwired: 1 in]
        n149 = call "Get Manager QueryErrors Request.vi"("gRPCid"=w556) -> ("error out"=w552:errorcluster, "Message Data"=w551:T58, "gRPCid out"=w555:T40)  [unwired: 8 in]
        n150 = Unbundle By Name(w551) -> ("query_all"=w550:bool)
        n151 = call "Get Errors.vi"("error in (no error)"=w552, "Parse All"=w550, "Plugin Manager in"=w553) -> ("error out"=w548:errorcluster, "Errors"=w547:T59[], "Plugin Manager out"=w549:refnum<class "CIFPluginManager.lvclass">)  [unwired: 6 in]
        n152 = for {
          tunnel: w547 -> [w566] mode=indexing
          tunnel: [w558] -> w545 mode=indexing
          n153 = Unbundle By Name(w566) -> ("error"=w564:bool, "code"=w563:i32, "Plugin"=w562:string, "Time"=w561:string, "Message"=w560:string, "Location"=w559:string)
          n154 = Bundle By Name(cluster=T15 {"error_status"=FALSE, "error_code"=0, "plugin"="", "time"="", "message"="", "location"=""} ("cif_manager_ErrorInfo"), "error_status"=w564, "error_code"=w563, "plugin"=w562, "time"=w561, "message"=w560, "location"=w559) -> (w558:T15)
        }
        n155 = Bundle By Name(cluster=T14 {"error_info"=[]} ("Message Data"), "error_info"=w545) -> (w544:T14)
        n156 = call "Set Manager QueryErrors Response.vi"("Message Data"=w544, "gRPCid in"=w555) -> ("error out"=w554:errorcluster)  [unwired: 9 in]
        n157 = Merge Errors(w548, w554) -> (w557:errorcluster)
      }
      event User Event {
        n158 = event-data() -> ("gRPCid"=w577:T40)  [unwired: 1 in]
        n159 = call "Get Manager QueryConfig Request.vi"("gRPCid"=w577) -> ("error out"=w571:errorcluster, "Message Data"=w576:T58, "gRPCid out"=w578:T40)  [unwired: 8 in]
        n160 = Unbundle By Name(w576) -> ("query_all"=w570:bool)
        n161 = call "Get Config Log.vi"("error in (no error)"=w571, "Parse All"=w570, "Plugin Manager in"=w572) -> ("error out"=w568:errorcluster, "Filtered Config Entries"=w567:string, "Plugin Manager out"=w569:refnum<class "CIFPluginManager.lvclass">)  [unwired: 6 in]
        n162 = Bundle By Name(cluster=T16 {"data"=""} ("Message Data"), "data"=w567) -> (w573:T16)
        n163 = call "Set Manager QueryConfig Response.vi"("Message Data"=w573, "gRPCid in"=w578) -> ("error out"=w575:errorcluster)  [unwired: 9 in]
        n164 = Merge Errors(w568, w575) -> (w579:errorcluster)
      }
      event User Event {
        n165 = event-data() -> ("gRPCid"=w590:T40)  [unwired: 1 in]
        n166 = call "Get Manager QueryInfo Request.vi"("gRPCid"=w590) -> ("error out"=w583:errorcluster, "Message Data"=w589:T58, "gRPCid out"=w588:T40)  [unwired: 8 in]
        n167 = Unbundle By Name(w589) -> ("query_all"=w584:bool)
        n168 = call "Get Info Log.vi"("error in (no error)"=w583, "Parse All"=w584, "Plugin Manager in"=w585) -> ("error out"=w582:errorcluster, "Filtered Info Entries"=w580:string, "Plugin Manager out"=w581:refnum<class "CIFPluginManager.lvclass">)  [unwired: 6 in]
        n169 = Bundle By Name(cluster=T16 {"data"=""} ("Message Data"), "data"=w580) -> (w586:T16)
        n170 = call "Set Manager QueryInfo Response.vi"("Message Data"=w586, "gRPCid in"=w588) -> ("error out"=w587:errorcluster)  [unwired: 9 in]
        n171 = Merge Errors(w582, w587) -> (w592:errorcluster)
      }
      event User Event {
        n172 = event-data() -> ("gRPCid"=w600:T40)  [unwired: 1 in]
        n173 = call "Get Manager ResetErrorIndex Request.vi"("gRPCid"=w600) -> ("error out"=w596:errorcluster, "gRPCid out"=w599:T40)  [unwired: 8 in, 1 out]
        n174 = case shown="No Error" w596 {
          selector: w596 -> [w605 w608]
          tunnel: w595 -> [w607 w609]
          tunnel: [w606 w609] -> w594
          tunnel: [w604 w608] -> w593
          frame No Error {
            n175 = call "Get Last Log Info.vi"("error in"=w605, "CIF Message Type"=Message_Type."Error") -> ("error out"=w604:errorcluster, "Log Info"=w602:T60)  [unwired: 8 in]
            n176 = Bundle By Name(cluster=w607, "Error Log Info"=w602) -> (w606:refnum<class "CIFPluginManager.lvclass">)
          }
          frame Error {
          }
        }
        n177 = call "Create Error Message.vi"("error in (no error)"=w593) -> ("Error Message"=w597:T57)  [unwired: 3 in]
        n178 = call "Set Manager ResetErrorIndex Response.vi"("Message Data"=w597, "gRPCid in"=w599) -> ("error out"=w598:errorcluster)  [unwired: 9 in]
        n179 = Merge Errors(w593, w598) -> (w601:errorcluster)
      }
      event User Event {
        n180 = event-data() -> ("gRPCid"=w614:T40)  [unwired: 1 in]
        n181 = call "Get Manager ResetConfigIndex Request.vi"("gRPCid"=w614) -> ("error out"=w613:errorcluster, "gRPCid out"=w612:T40)  [unwired: 8 in, 1 out]
        n182 = case shown="No Error" w613 {
          selector: w613 -> [w621 w625]
          tunnel: w617 -> [w624 w626]
          tunnel: [w623 w626] -> w616
          tunnel: [w620 w625] -> w615
          frame No Error {
            n183 = call "Get Last Log Info.vi"("error in"=w621, "CIF Message Type"=Message_Type."Configuration") -> ("error out"=w620:errorcluster, "Log Info"=w619:T60)  [unwired: 8 in]
            n184 = Bundle By Name(cluster=w624, "Config Log Info"=w619) -> (w623:refnum<class "CIFPluginManager.lvclass">)
          }
          frame Error {
          }
        }
        n185 = call "Create Error Message.vi"("error in (no error)"=w615) -> ("Error Message"=w610:T57)  [unwired: 3 in]
        n186 = call "Set Manager ResetConfigIndex Response.vi"("Message Data"=w610, "gRPCid in"=w612) -> ("error out"=w611:errorcluster)  [unwired: 9 in]
        n187 = Merge Errors(w615, w611) -> (w618:errorcluster)
      }
      event User Event {
        n188 = event-data() -> ("gRPCid"=w634:T40)  [unwired: 1 in]
        n189 = call "Get Manager ResetInfoIndex Request.vi"("gRPCid"=w634) -> ("error out"=w629:errorcluster, "gRPCid out"=w631:T40)  [unwired: 8 in, 1 out]
        n190 = case shown="No Error" w629 {
          selector: w629 -> [w638 w642]
          tunnel: w630 -> [w641 w643]
          tunnel: [w640 w643] -> w628
          tunnel: [w637 w642] -> w627
          frame No Error {
            n191 = call "Get Last Log Info.vi"("error in"=w638, "CIF Message Type"=Message_Type."Information") -> ("error out"=w637:errorcluster, "Log Info"=w636:T60)  [unwired: 8 in]
            n192 = Bundle By Name(cluster=w641, "Info Log Info"=w636) -> (w640:refnum<class "CIFPluginManager.lvclass">)
          }
          frame Error {
          }
        }
        n193 = call "Create Error Message.vi"("error in (no error)"=w627) -> ("Error Message"=w632:T57)  [unwired: 3 in]
        n194 = call "Set Manager ResetInfoIndex Response.vi"("Message Data"=w632, "gRPCid in"=w631) -> ("error out"=w633:errorcluster)  [unwired: 9 in]
        n195 = Merge Errors(w627, w633) -> (w635:errorcluster)
      }
      event User Event {
        n196 = event-data() -> ("gRPCid"=w653:T40)  [unwired: 1 in]
        n197 = call "Get Manager QueryPluginInfo Request.vi"("gRPCid"=w653) -> ("error out"=w645:errorcluster, "gRPCid out"=w652:T40)  [unwired: 8 in, 1 out]
        n198 = call "Get Plugin Map.vi"("error in (no error)"=w645, "CIFPluginManager in"=w647) -> ("error out"=w644:errorcluster, "Plugin Map"=w646:T42)  [unwired: 8 in]
        n199 = for {
          tunnel: w646 -> [w667] mode=indexing
          tunnel: [w662] -> w649 mode=indexing
          n200 = Unbundle By Name(w667) -> ("Plugin Management Data.status"=w658:T19, "Unique Name"=w665:string, "Plugin Management Data.Plugin Type"=w664:string, "Plugin Management Data.gRPC Port"=w663:i32, "Plugin Management Data.Version.Major"=w659:i32, "Plugin Management Data.Version.Minor"=w660:i32, "Plugin Management Data.Version.Fix"=w661:i32)
          n201 = To Unsigned Long Integer(number=w659) -> (unsigned 32bit integer=w657:u32)
          n202 = To Unsigned Long Integer(number=w660) -> (unsigned 32bit integer=w656:u32)
          n203 = To Unsigned Long Integer(number=w661) -> (unsigned 32bit integer=w655:u32)
          n204 = Bundle By Name(cluster=T18 {"plugin_name"="", "plugin_type"="", "grpc_port"=0, "plugin_version"={"major"=0, "minor"=0, "fix"=0}, "status"={"state"=enum."PLUGINSTATE_UNKNOWN", "timing_statistics"={"period"={"max"=0, "min"=0, "avg"=0.0}, "wake_error"={"max"=0, "min"=0, "avg"=0.0}, "execute"={"max"=0, "min"=0, "avg"=0.0}, "housekeep"={"max"=0, "min"=0, "avg"=0.0}, "idle"={"max"=0, "min"=0, "avg"=0.0}, "cleanup"={"max"=0, "min"=0, "avg"=0.0}, "custom_1"={"max"=0, "min"=0, "avg"=0.0}, "custom_2"={"max"=0, "min"=0, "avg"=0.0}}, "fifo_statistics"={"from_t0"={"max"=0, "min"=0, "avg"=0.0}, "from_previous_plugin"={"max"=0, "min"=0, "avg"=0.0}, "output_error"={"max"=0, "min"=0, "avg"=0.0}}, "error"={"status"=FALSE, "code"=0}, "monitor_doubles"={"double_1"=0.0, "double_2"=0.0, "double_3"=0.0, "double_4"=0.0}, "monitor_u64s"={"u64_1"=0, "u64_2"=0, "u64_3"=0, "u64_4"=0}, "monitor_i64s"={"i64_1"=0, "i64_2"=0, "i64_3"=0, "i64_4"=0}}, "loader_info"={"loader_type"=enum."LOADERTYPE_UNKNOWN", "loader_name"=""}} ("cif_manager_PluginInfo"), "status"=w658, "plugin_name"=w665, "plugin_type"=w664, "grpc_port"=w663, "plugin_version.major"=w657, "plugin_version.minor"=w656, "plugin_version.fix"=w655) -> (w662:T18)
        }
        n205 = Bundle By Name(cluster=T17 {"plugin_info"=[]} ("Message Data"), "plugin_info"=w649) -> (w648:T17)
        n206 = call "Set Manager QueryPluginInfo Response.vi"("Message Data"=w648, "gRPCid in"=w652) -> ("error out"=w651:errorcluster)  [unwired: 9 in]
        n207 = Merge Errors(w644, w651) -> (w654:errorcluster)
      }
      event User Event {
        # "Don't log query error to main log, only pass to gRPC client."
        n208 = event-data() -> ("gRPCid"=w696:T40)  [unwired: 1 in]
        n209 = call "Get Manager QueryPlugin Request.vi"("gRPCid"=w696) -> ("error out"=w674:errorcluster, "Message Data"=w691:T61, "gRPCid out"=w695:T40)  [unwired: 8 in]
        n210 = Unbundle By Name(w691) -> ("plugin_name"=w681:string)
        n211 = call "Get Plugin Map.vi"("error in (no error)"=w674, "CIFPluginManager in"=w676) -> ("error out"=w673:errorcluster, "Plugin Map"=w675:T42)  [unwired: 8 in]
        n212 = Look In Map(map=w675, key=w681) -> (key not found?=w680:bool, value=w690:T43)  [unwired: 1 in]
        n213 = call <vilib>:"Add Error.vi"("error in (no error)"=w673, "String to Append"=w681, "Error"=Errors."Plugin Not Found", "Insert Error"=w680) -> ("error out"=w682:errorcluster)  [unwired: 7 in]
        n214 = Unbundle By Name(w690) -> ("Loader Type"=w671:T44, "Loader"=w672:string, "status"=w668:T19, "Unique Name"=w669:string, "Plugin Type"=w693:string, "gRPC Port"=w692:i32, "Version.Major"=w688:i32, "Version.Minor"=w686:i32, "Version.Fix"=w687:i32)
        n215 = call "Create Error Message.vi"("error in (no error)"=w682) -> ("Error Message"=w685:T57)  [unwired: 3 in]
        n216 = To Unsigned Long Integer(number=w688) -> (unsigned 32bit integer=w679:u32)
        n217 = To Unsigned Long Integer(number=w686) -> (unsigned 32bit integer=w678:u32)
        n218 = To Unsigned Long Integer(number=w687) -> (unsigned 32bit integer=w677:u32)
        n219 = call "Convert Loader Type to gRPC Type.vi"("Loader Type"=w671) -> ("Loader Type"=w670:T29)  [unwired: 10 in]
        n220 = Bundle By Name(cluster=T31 {"plugin_info"={"plugin_name"="", "plugin_type"="", "grpc_port"=0, "plugin_version"={"major"=0, "minor"=0, "fix"=0}, "status"={"state"=enum."PLUGINSTATE_UNKNOWN", "timing_statistics"={"period"={"max"=0, "min"=0, "avg"=0.0}, "wake_error"={"max"=0, "min"=0, "avg"=0.0}, "execute"={"max"=0, "min"=0, "avg"=0.0}, "housekeep"={"max"=0, "min"=0, "avg"=0.0}, "idle"={"max"=0, "min"=0, "avg"=0.0}, "cleanup"={"max"=0, "min"=0, "avg"=0.0}, "custom_1"={"max"=0, "min"=0, "avg"=0.0}, "custom_2"={"max"=0, "min"=0, "avg"=0.0}}, "fifo_statistics"={"from_t0"={"max"=0, "min"=0, "avg"=0.0}, "from_previous_plugin"={"max"=0, "min"=0, "avg"=0.0}, "output_error"={"max"=0, "min"=0, "avg"=0.0}}, "error"={"status"=FALSE, "code"=0}, "monitor_doubles"={"double_1"=0.0, "double_2"=0.0, "double_3"=0.0, "double_4"=0.0}, "monitor_u64s"={"u64_1"=0, "u64_2"=0, "u64_3"=0, "u64_4"=0}, "monitor_i64s"={"i64_1"=0, "i64_2"=0, "i64_3"=0, "i64_4"=0}}, "loader_info"={"loader_type"=enum."LOADERTYPE_UNKNOWN", "loader_name"=""}}, "status"={"code"=0, "message"=""}} ("Message Data"), "plugin_info.loader_info.loader_type"=w670, "plugin_info.loader_info.loader_name"=w672, "plugin_info.status"=w668, "plugin_info.plugin_name"=w669, "plugin_info.plugin_type"=w693, "plugin_info.grpc_port"=w692, "plugin_info.plugin_version.major"=w679, "plugin_info.plugin_version.minor"=w678, "plugin_info.plugin_version.fix"=w677, "status"=w685) -> (w684:T31)
        n221 = call "Set Manager QueryPlugin Response.vi"("Message Data"=w684, "gRPCid in"=w695) -> ("error out"=w694:errorcluster)  [unwired: 9 in]
        n222 = Merge Errors(w673, w694) -> (w697:errorcluster)
      }
      event User Event {
        n223 = event-data() -> ("gRPCid"=w705:T40)  [unwired: 1 in]
        n224 = call "Get Manager QueryClockStatus Request.vi"("gRPCid"=w705) -> ("error out"=w699:errorcluster, "gRPCid out"=w707:T40)  [unwired: 8 in, 1 out]
        n225 = call "Get Clock History Map.vi"("error in (no error)"=w699, "CIFPluginManager in"=w701) -> ("error out"=w698:errorcluster, "Clock History Map"=w700:T62)  [unwired: 8 in]
        n226 = call <vilib>:"Clock Map to Clock Array.vi"("error in (no error)"=w698, "Clock History Map in"=w700) -> ("error out"=w709:errorcluster, "Clock Conversion Array"=w708:T64[], "Clock History Map out"=w702:T62)  [unwired: 7 in]
        n227 = for {
          tunnel: w708 -> [w725] mode=indexing
          tunnel: [w718] -> w710 mode=indexing
          tunnel: w702 -> [w716]
          n228 = Unbundle By Name(w725) -> ("ClockID"=w715:u8, "Last Reset"=w719:i64, "Offset Pair.System Time"=w720:i64, "Offset Pair.External Time"=w721:i64, "Slope"=w722:dbl, "Name"=w723:string)
          n229 = To Unsigned Long Integer(number=w715) -> (unsigned 32bit integer=w724:u32)
          n230 = call <vilib>:"Calculate Error.vi"("ClockID"=w715, "Clock History Map in"=w716) -> ("Error Statistics (ns)"=w714:T65)  [unwired: 8 in, 1 out]
          n231 = Unbundle By Name(w714) -> ("mean"=w713:i64, "standard deviation"=w712:i64)
          n232 = Bundle By Name(cluster=T34 {"clock_conversion"={"clock_id"=0, "last_reset"=0, "slope"=0.0, "offset_pair"={"system_time"=0, "external_time"=0}, "clock_name"=""}, "error_mean"=0, "error_std_dev"=0} ("cif_manager_ClockStatus"), "error_mean"=w713, "error_std_dev"=w712, "clock_conversion.clock_id"=w724, "clock_conversion.last_reset"=w719, "clock_conversion.offset_pair.system_time"=w720, "clock_conversion.offset_pair.external_time"=w721, "clock_conversion.slope"=w722, "clock_conversion.clock_name"=w723) -> (w718:T34)
        }
        n233 = Bundle By Name(cluster=T33 {"clocks_status"=[]} ("Message Data"), "clocks_status"=w710) -> (w703:T33)
        n234 = call "Set Manager QueryClockStatus Response.vi"("Message Data"=w703, "gRPCid in"=w707) -> ("error out"=w706:errorcluster)  [unwired: 9 in]
        n235 = Merge Errors(w709, w706) -> (w711:errorcluster)
      }
      event User Event {
        # "Could add clock log function"
        n236 = event-data() -> ("gRPCid"=w736:T40)  [unwired: 1 in]
        n237 = call "Get Manager UpdateClock Request.vi"("gRPCid"=w736) -> ("error out"=w732:errorcluster, "Message Data"=w731:T66, "gRPCid out"=w735:T40)  [unwired: 8 in]
        n238 = Unbundle By Name(w730) -> ("Clock History Map DVR"=w729:refnum<data-value>)
        n239 = in-place {
          in-place-border: [w752] -> w728
          in-place-border: w732 -> [w740]
          in-place-border: w731 -> [w751]
          n240 = in-place-dvr #9(w729) -> (w742:T62, w739:errorcluster)
          n241 = Merge Errors(w740, w739) -> (w738:errorcluster)
          n242 = Unbundle By Name(w751) -> ("timestamp_pair.system_time"=w745:i64, "timestamp_pair.external_time"=w744:i64, "reinit"=w747:bool, "clock_id"=w750:u32, "clock_name"=w749:string)
          n243 = Bundle By Name(cluster=T37 {"System Time"=0, "External Time"=0} ("Timestamp Pair"), "System Time"=w745, "External Time"=w744) -> (w743:T37)
          n244 = To Unsigned Byte Integer(number=w750) -> (unsigned 8bit integer=w748:u8)
          n245 = call <vilib>:"Update Clock Map.vi"("Name"=w749, "Reset"=w747, "error in (no error)"=w738, "ClockID"=w748, "Timestamp Pair"=w743, "Clock History Map in"=w742) -> ("error out"=w752:errorcluster, "Clock History Map out"=w741:map{u8, T63})  [unwired: 4 in]
          n246 = in-place-dvr #9(w741) -> (w727:errorcluster)  [unwired: 1 out]
        }
        n247 = Merge Errors(w728, w727) -> (w726:errorcluster)
        n248 = call "Create Error Message.vi"("error in (no error)"=w726) -> ("Error Message"=w733:T57)  [unwired: 3 in]
        n249 = call "Set Manager UpdateClock Response.vi"("Message Data"=w733, "gRPCid in"=w735) -> ("error out"=w734:errorcluster)  [unwired: 9 in]
        n250 = Merge Errors(w726, w734) -> (w737:errorcluster)
      }
      event User Event {
        n251 = event-data() -> ("gRPCid"=w784:T40)  [unwired: 1 in]
        n252 = call "Get Manager CreateOrch Request.vi"("gRPCid"=w784) -> ("error out"=w779:errorcluster, "Message Data"=w778:T67, "gRPCid out"=w783:T40)  [unwired: 8 in]
        n253 = Unbundle By Name(w778) -> ("start_timestamp"=w755:u64, "filename"=w773:string, "default_ip"=w774:string, "orchestration_language"=w769:T68, "create_file"=w768:bool)
        n254 = To Quad Integer(1:w755) -> (0:w753:i64)
        n255 = call <vilib>:"TAI Time to LabVIEW Time.vi"("TAI Time (ns)"=w753) -> ("LabVIEW Time (s)"=w756:timestamp)  [unwired: 4 in]
        n256 = Not Equal To 0?(x=w755) -> (x != 0?=w777:bool)
        n257 = call <vilib>:"Trim Whitespace.vi"("string"=w773) -> ("trimmed string"=w759:string)  [unwired: 1 in]
        n258 = call <vilib>:"Trim Whitespace.vi"("string"=w774) -> ("trimmed string"=w772:string)  [unwired: 1 in]
        n259 = Format Date/Time String(time format string (%c)="%m/%d/%Y %H:%M:%S", seconds (now)=w756, UTC format=TRUE) -> (date/time string=w754:string)
        n260 = call "Get Config Log.vi"("Parse Timestamp"=w754, "error in (no error)"=w779, "Parse All"=w777, "Plugin Manager in"=w781) -> ("error out"=w775:errorcluster, "Filtered Config Entries"=w776:string, "Plugin Manager out"=w780:refnum<class "CIFPluginManager.lvclass">)  [unwired: 5 in]
        n261 = Empty String/Path?(string/path=w772) -> (empty?=w771:bool)
        n262 = Not(x=w771) -> (.not. x?=w770:bool)
        n263 = case shown="\"ORCHESTRATIONLANGUAGE_PYTHON\", Default" w769 {
          tunnel: w776 -> [w798]
          tunnel: w775 -> [w797]
          tunnel: w759 -> [w796]
          tunnel: w772 -> [w795]
          tunnel: w770 -> [w794]
          tunnel: [w793] -> w766
          tunnel: [w792] -> w767
          tunnel: [w791] -> w760
          frame "ORCHESTRATIONLANGUAGE_PYTHON", Default {
            n264 = call "Create Python Orchestration Script.vi"("Override Address"=w794, "error in"=w797, "Default Address"=w795, "Configuration File Name"=w796, "Filtered Config Entries"=w798) -> ("error out"=w793:errorcluster, "Orchestration File Path"=w792:path, "Python Orchestration File"=w791:string)  [unwired: 4 in]
          }
        }
        n265 = case shown="True" w768 {
          tunnel: w760 -> [_ w788]
          tunnel: w767 -> [_ w789]
          tunnel: w766 -> [w786 w790]
          tunnel: [w786 w787] -> w763
          frame False {
          }
          frame True {
            n266 = Write to Text File(file (use dialog)=w789, text=w788, error in=w790) -> (error out=w787:errorcluster)  [unwired: 1 in, 2 out]
          }
        }
        n267 = call "Create Error Message.vi"("error in (no error)"=w763) -> ("Error Message"=w764:T57)  [unwired: 3 in]
        n268 = Bundle By Name(cluster=T38 {"orchestration_script"="", "status"={"code"=0, "message"=""}} ("Message Data"), "status"=w764) -> (w762:T38)
        n269 = Bundle By Name(cluster=w762, "orchestration_script"=w760) -> (w761:T38)
        n270 = call "Set Manager CreateOrch Response.vi"("Message Data"=w761, "gRPCid in"=w783) -> ("error out"=w782:errorcluster)  [unwired: 9 in]
        n271 = Merge Errors(w763, w782) -> (w785:errorcluster)
      }
      event User Event {
        # "Ignore socket closed error"
        # "For faster UI don't wait on loader to respond"
        n272 = event-data() -> ("gRPCid"=w812:T40)  [unwired: 1 in]
        n273 = call "Get Manager DestroyPluginLoader Request.vi"("gRPCid"=w812) -> ("error out"=w806:errorcluster, "Message Data"=w808:T69, "gRPCid out"=w811:T40)  [unwired: 8 in]
        n274 = Unbundle By Name(w808) -> ("loader_name"=w805:string)
        n275 = call "Request Plugin Loader Stop.vi"("error in (no error)"=w806, "Plugin Loader Name"=w805, "CIFPluginManager in"=w807) -> ("error out"=w802:errorcluster, "gRPC ID"=w804:T40)  [unwired: 7 in]
        n276 = call "Destroy Loader.vi"("error in"=w802, "gRPC ID in"=w804) -> ("error out"=w803:errorcluster)  [unwired: 8 in, 1 out]
        n277 = call <vilib>:"Clear Errors.vi"("error in (no error)"=w803, "specific error code to clear (0: all)"=-1014) -> ("error out"=w809:errorcluster)  [unwired: 4 in, 1 out]
        n278 = call "Create Error Message.vi"("error in (no error)"=w802) -> ("Error Message"=w800:T57)  [unwired: 3 in]
        n279 = Bundle By Name(cluster=T39 {"status"={"code"=0, "message"=""}} ("Message Data"), "status"=w800) -> (w799:T39)
        n280 = call "Set Manager DestroyPluginLoader Response.vi"("Message Data"=w799, "gRPCid in"=w811) -> ("error out"=w810:errorcluster)  [unwired: 9 in]
        n281 = Merge Errors(w809, w810) -> (w814:errorcluster)
      }
      event User Event {
        n282 = event-data() -> ()  [unwired: 1 in, 2 out]
        n283 = Unbundle By Name(w816) -> ("Shutdown"=w817:refnum<user-event>)
        n284 = Generate User Event(user event=w817, event data cluster=TRUE ("event data")) -> ()  [unwired: 2 in, 2 out]
      }
    }
    n285 = call "Filter and Log Error.vi"("error In"=w13, "Name"=w9) -> ()  [unwired: 10 in]
  }
  "Plugin Manager out" <- w5
  n286 = Unregister For Events(event registration refnum=w6) -> (error out=→"error out":errorcluster)  [unwired: 1 in]
